vi "Autonomous IndependentAPRIL1st.vi"() -> ()   [LabVIEW 2016]
doc: "This VI is called when autonomous begins, and will automatically be terminated when autonomous ends. You can carry out timed or sensor driven robot movement independently without needing to return to the caller."
uses:
  <vilib>/Rock Robotics/WPI/Utilities/WPI_GetSetVariantRefNum.vi
  <vilib>/Rock Robotics/Network Tables/NT Read String.vi
  <vilib>/Rock Robotics/Network Tables/NT Write Numeric Array.vi
  <vilib>/Rock Robotics/WPI/RobotDrive/WPI_RobotDriveArcadeDrive_Standard(NoSaturation).vi
  <vilib>/Rock Robotics/Network Tables/NT Read Boolean.vi
  <vilib>/Rock Robotics/Network Tables/NT Write Number.vi
  Robot Global Data.vi
  <vilib>/Rock Robotics/WPI/Counter/WPI_CounterDigitalInputToDigitalSource.vi
  <vilib>/Rock Robotics/SystemInterfaces/DIO/FPGA_DIOChannel.ctl
panel:
  out "Hook Center Cons":dbl
  out "gyro":dbl
  out "sonar distance (inches)":dbl
  out "Encoder Loop":dbl
  out "Encoder Loop":string
  out "Current Movement, for debugging 2":T1 {"Y Joystick Value" scale=1.0..-1.0; "X Joystick Value" scale=-1.0..1.0}
  in  "Array of robot movements 2":T2(array[cluster])=[{"X Joystick Value"=0.39393939393939403, "Y Joystick Value"=0.0, "Delay (sec)"=1.0, "Movement Name"="turn"}, {"X Joystick Value"=-0.3737373737373737, "Y Joystick Value"=0.0, "Delay (sec)"=1.0, "Movement Name"="turn back"}] {"Y Joystick Value" scale=1.0..-1.0; "X Joystick Value" scale=-1.0..1.0}
  out "Current Movement, for debugging":T1 {"Y Joystick Value" scale=1.0..-1.0; "X Joystick Value" scale=-1.0..1.0}
  in  "Array of robot movements":T2(array[cluster])=[{"X Joystick Value"=0.39393939393939403, "Y Joystick Value"=0.0, "Delay (sec)"=1.0, "Movement Name"="turn"}, {"X Joystick Value"=-0.3737373737373737, "Y Joystick Value"=0.0, "Delay (sec)"=1.0, "Movement Name"="turn back"}] {"Y Joystick Value" scale=1.0..-1.0; "X Joystick Value" scale=-1.0..1.0}
  # "Sensor Readings\nConstanly updated in\nwhile loopes"
  # "Be sure to right-click and choose Data Operations>>Make Current Value default if you want to save the array values with the VI"
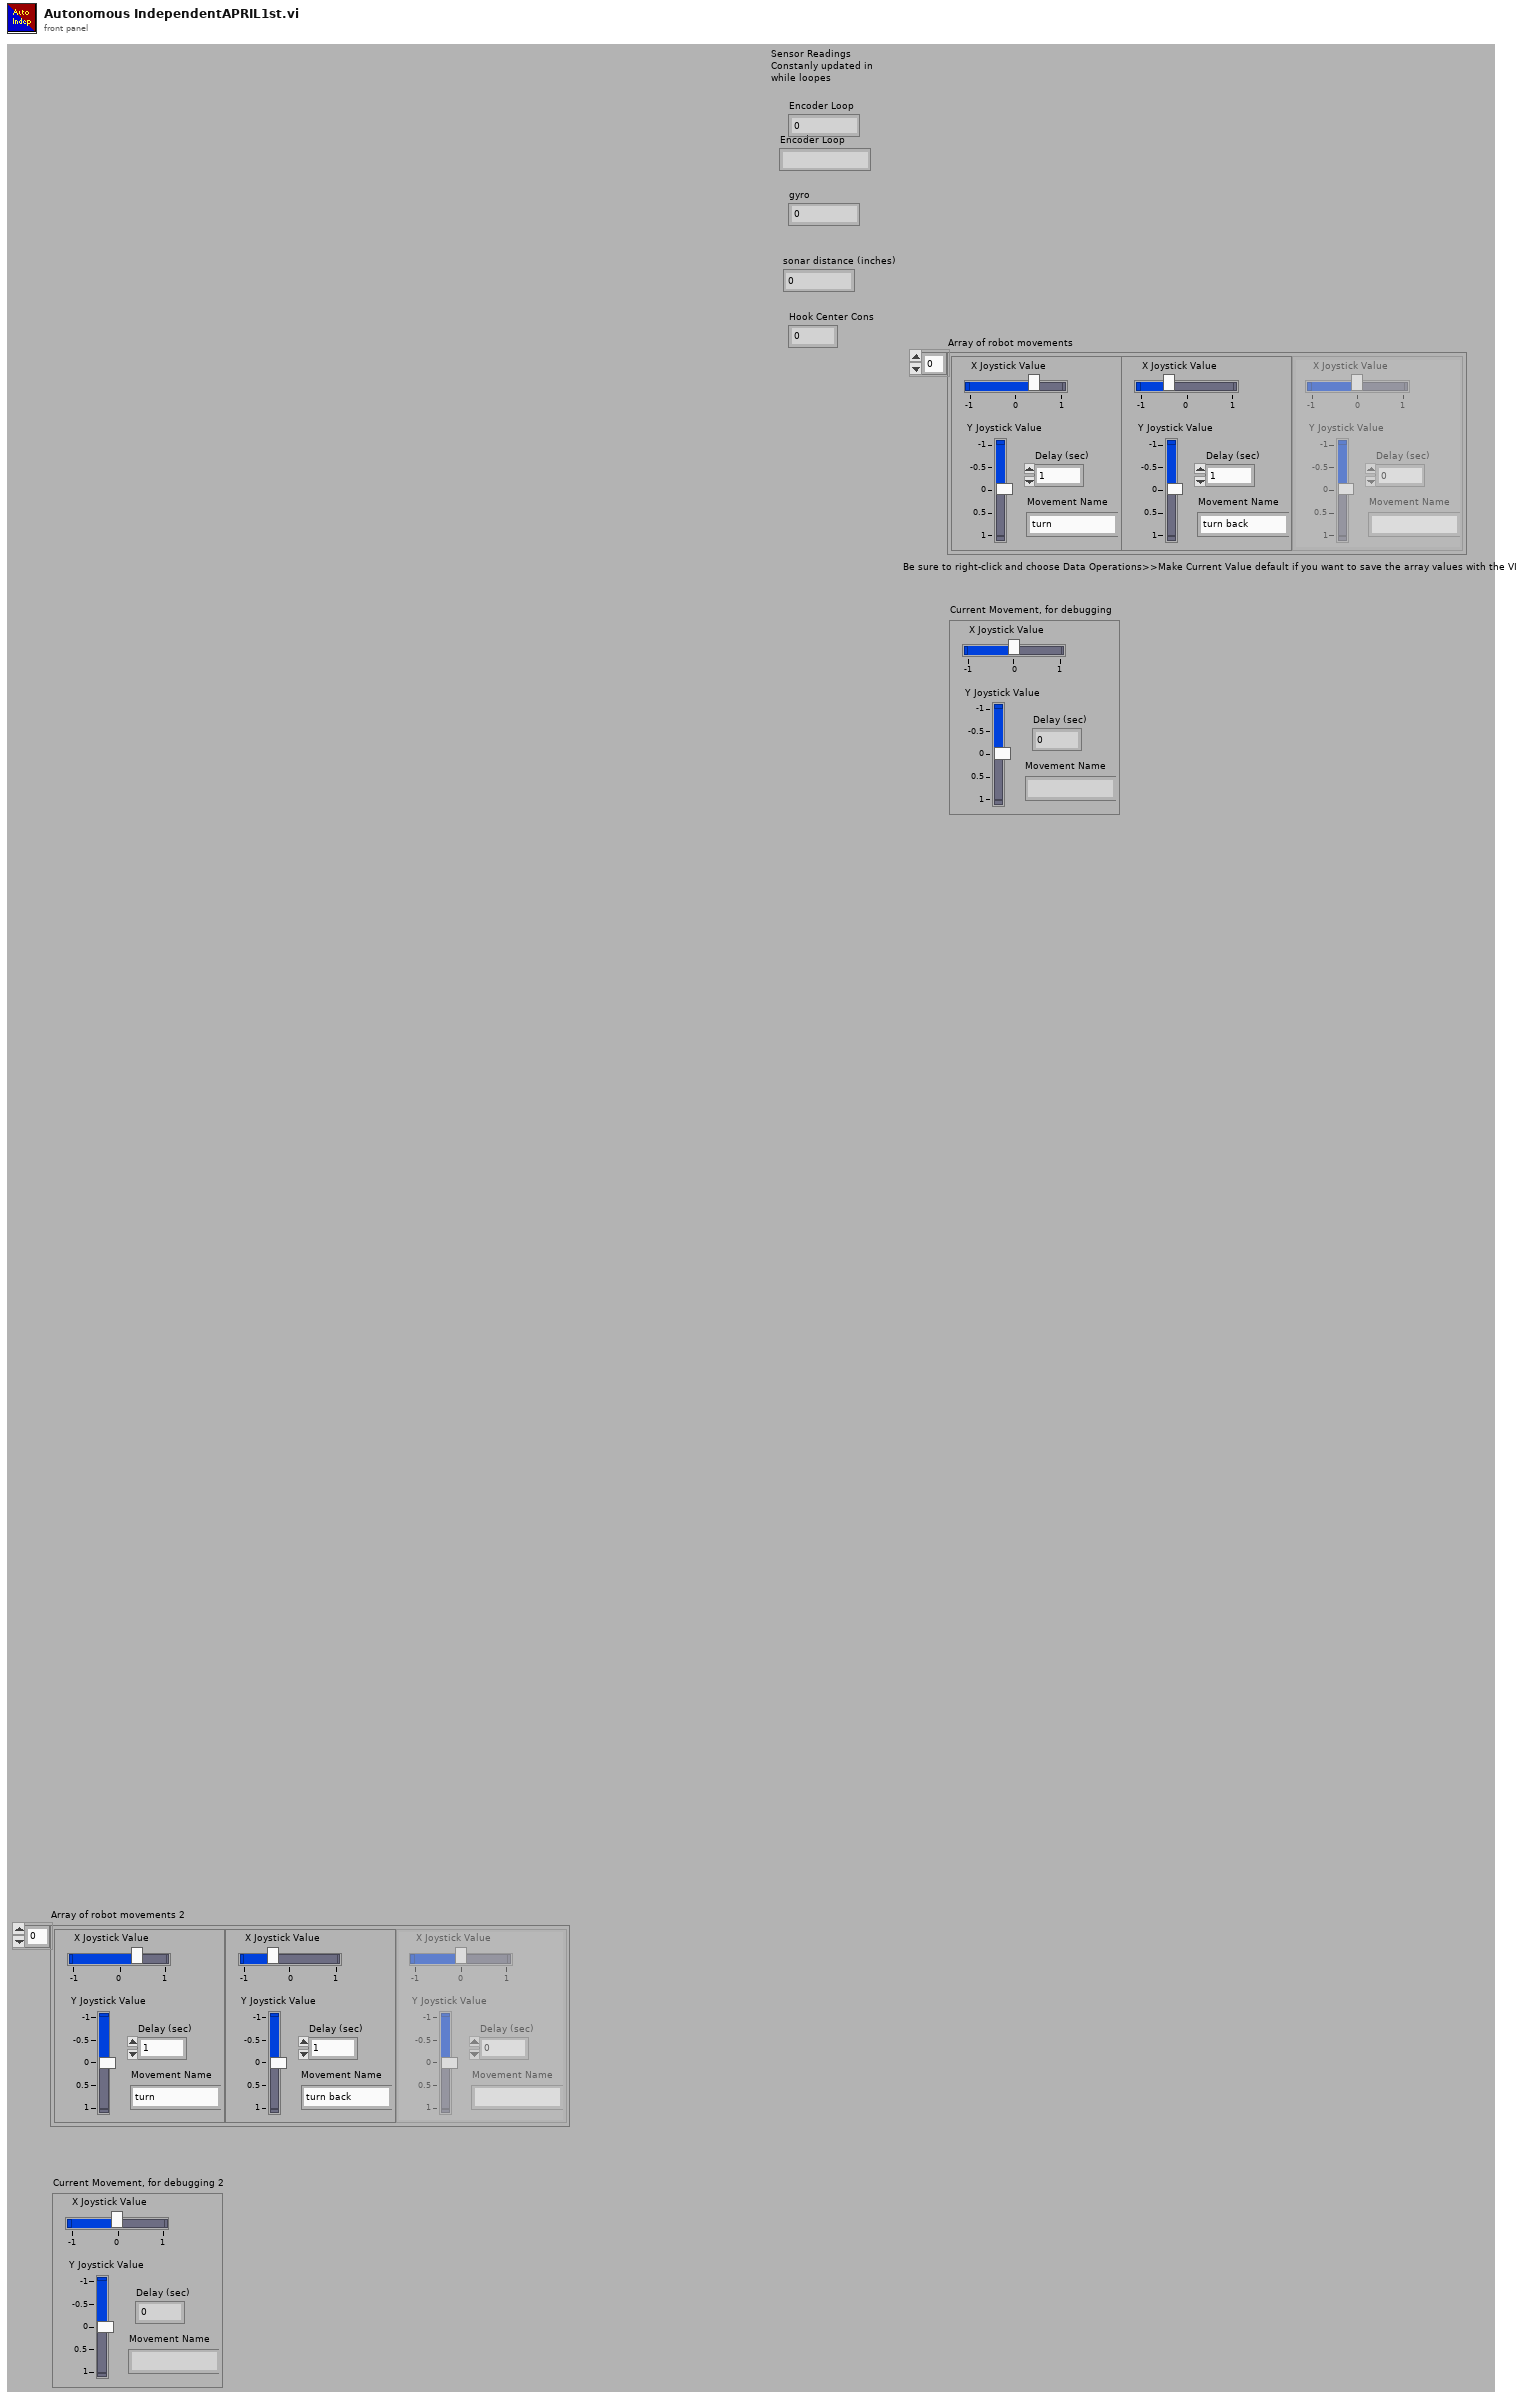
[diagram p1: front panel]
types:
  T1 = cluster{"X Joystick Value":dbl, "Y Joystick Value":dbl, "Delay (sec)":dbl, "Movement Name":string}
  T2 = cluster{"X Joystick Value":dbl, "Y Joystick Value":dbl, "Delay (sec)":dbl, "Movement Name":string}[]
  T3 = typedef "FPGA_DIOChannel.ctl" = enum8{"DIO 0", "DIO 1", "DIO 2", "DIO 3", "DIO 4", "DIO 5", "DIO 6", "DIO 7", "DIO 8", "DIO 9", "DIO MXP 0", "DIO MXP 1", "DIO MXP 2", "DIO MXP 3", "DIO MXP 4", "DIO MXP 5", "DIO MXP 6", "DIO MXP 7", "DIO MXP 8", "DIO MXP 9", "DIO MXP 10", "DIO MXP 11", "DIO MXP 12", "DIO MXP 13", "DIO MXP 14", "DIO MXP 15", "SPI Port CS1", "SPI Port CS2", "SPI Port CS3", "SPI Port MISO", "SPI Port MOSI", "Invalid"}
  T4 = typedef "WPI_DigitalInputDevRef.ctl" = cluster{"DevStatus":errorcluster, "DIO Channel":T3}
  T5 = typedef "FPGA_CounterEncoderSourceConvertionLVSourceType.ctl" = cluster{"DevStatus":errorcluster, "AnalogTriggerMode?":bool, "DigitalMode":cluster{"DIO Channel":T6}, "AnalogTriggerMode":cluster{"AnalogTriggerIndex":T7, "OutputType":T8}}
  T6 = typedef "FPGA_DIODigitalSourceChannel.ctl" = enum8{"DIO 0", "DIO 1", "DIO 2", "DIO 3", "DIO 4", "DIO 5", "DIO 6", "DIO 7", "DIO 8", "DIO 9", "DIO MXP 0", "DIO MXP 1", "DIO MXP 2", "DIO MXP 3", "DIO MXP 4", "DIO MXP 5", "DIO MXP 6", "DIO MXP 7", "DIO MXP 8", "DIO MXP 9", "DIO MXP 10", "DIO MXP 11", "DIO MXP 12", "DIO MXP 13", "DIO MXP 14", "DIO MXP 15", "Disabled"}
  T7 = typedef "FPGA_AnalogTriggerIndex.ctl" = enum8{"Trig 0", "Trig 1", "Trig 2", "Trig 3", "Trig 4", "Trig 5", "Trig 6", "Trig 7", "Invalid"}
  T8 = typedef "FPGA_AnalogTriggerOutType.ctl" = enum16{"InWindow", "TriggerState", "Rising", "Falling"}
  T9 = typedef "WPI_EncoderDevRef.ctl" = cluster{"DevStatus":errorcluster, "EncoderIndex":T10, "CounterIndex":T11, "DistancePerCount":dbl, "Decoding Type":T12}
  T10 = typedef "FPGA_EncoderIdx.ctl" = enum8{"Enc 0", "Enc 1", "Enc 2", "Enc 3", "Enc 4", "Enc 5", "Enc 6", "Enc 7", "Invalid"}
  T11 = typedef "FPGA_CounterCtrSystemIndex.ctl" = enum8{"Ctr 0", "Ctr 1", "Ctr 2", "Ctr 3", "Ctr 4", "Ctr 5", "Ctr 6", "Ctr 7", "Invalid"}
  T12 = typedef "WPI_EncoderType.ctl" = enum16{"1x", "2x", "4x"}
  T13 = typedef "WPI_JoystickDevRef.ctl" = cluster{"Device":T14}
  T14 = typedef "WPI_JoystickDeviceEnum.ctl" = enum16{"USB 0", "USB 1", "USB 2", "USB 3", "USB 4", "USB 5"}
  T15 = typedef "WPI_DriverStationPositionInfo.ctl" = enum16{"1", "2", "3"}
  T16 = typedef "WPI_RobotDriveDevRef.ctl" = cluster{"DevStatus":errorcluster, "Motors[]":T17[], "Square Inputs":bool, "Max Output":dbl}
  T17 = typedef "WPI_MotorControlDeviceRef.ctl" = cluster{"DeviceStatus":errorcluster, "Type":T18, "PWM":cluster{"PWM Channel":T19, "DeadBand":T20}, "CAN":cluster{"Device Number":u8, "SetOutput VI Ref":variant, "GetOutput VI Ref":variant, "Enable VI Ref":variant, "Disable VI Ref":variant, "Data":variant}, "Invert":bool}
  T18 = typedef "WPI_MotorControlType.ctl" = enum16{"PWM", "CAN"}
  T19 = typedef "FPGA_DIOPWMChannel.ctl" = enum8{"PWM 0", "PWM 1", "PWM 2", "PWM 3", "PWM 4", "PWM 5", "PWM 6", "PWM 7", "PWM 8", "PWM 9", "PWM MXP 0", "PWM MXP 1", "PWM MXP 2", "PWM MXP 3", "PWM MXP 4", "PWM MXP 5", "PWM MXP 6", "PWM MXP 7", "PWM MXP 8", "PWM MXP 9", "Invalid"}
  T20 = typedef "WPI_PWMDeadband.ctl" = cluster{"Name":string, "maxPositivePwm":i32, "minPositivePwm":i32, "centerPwm":i32, "maxNegativePwm":i32, "minNegativePwm":i32, "angularRange":u16}
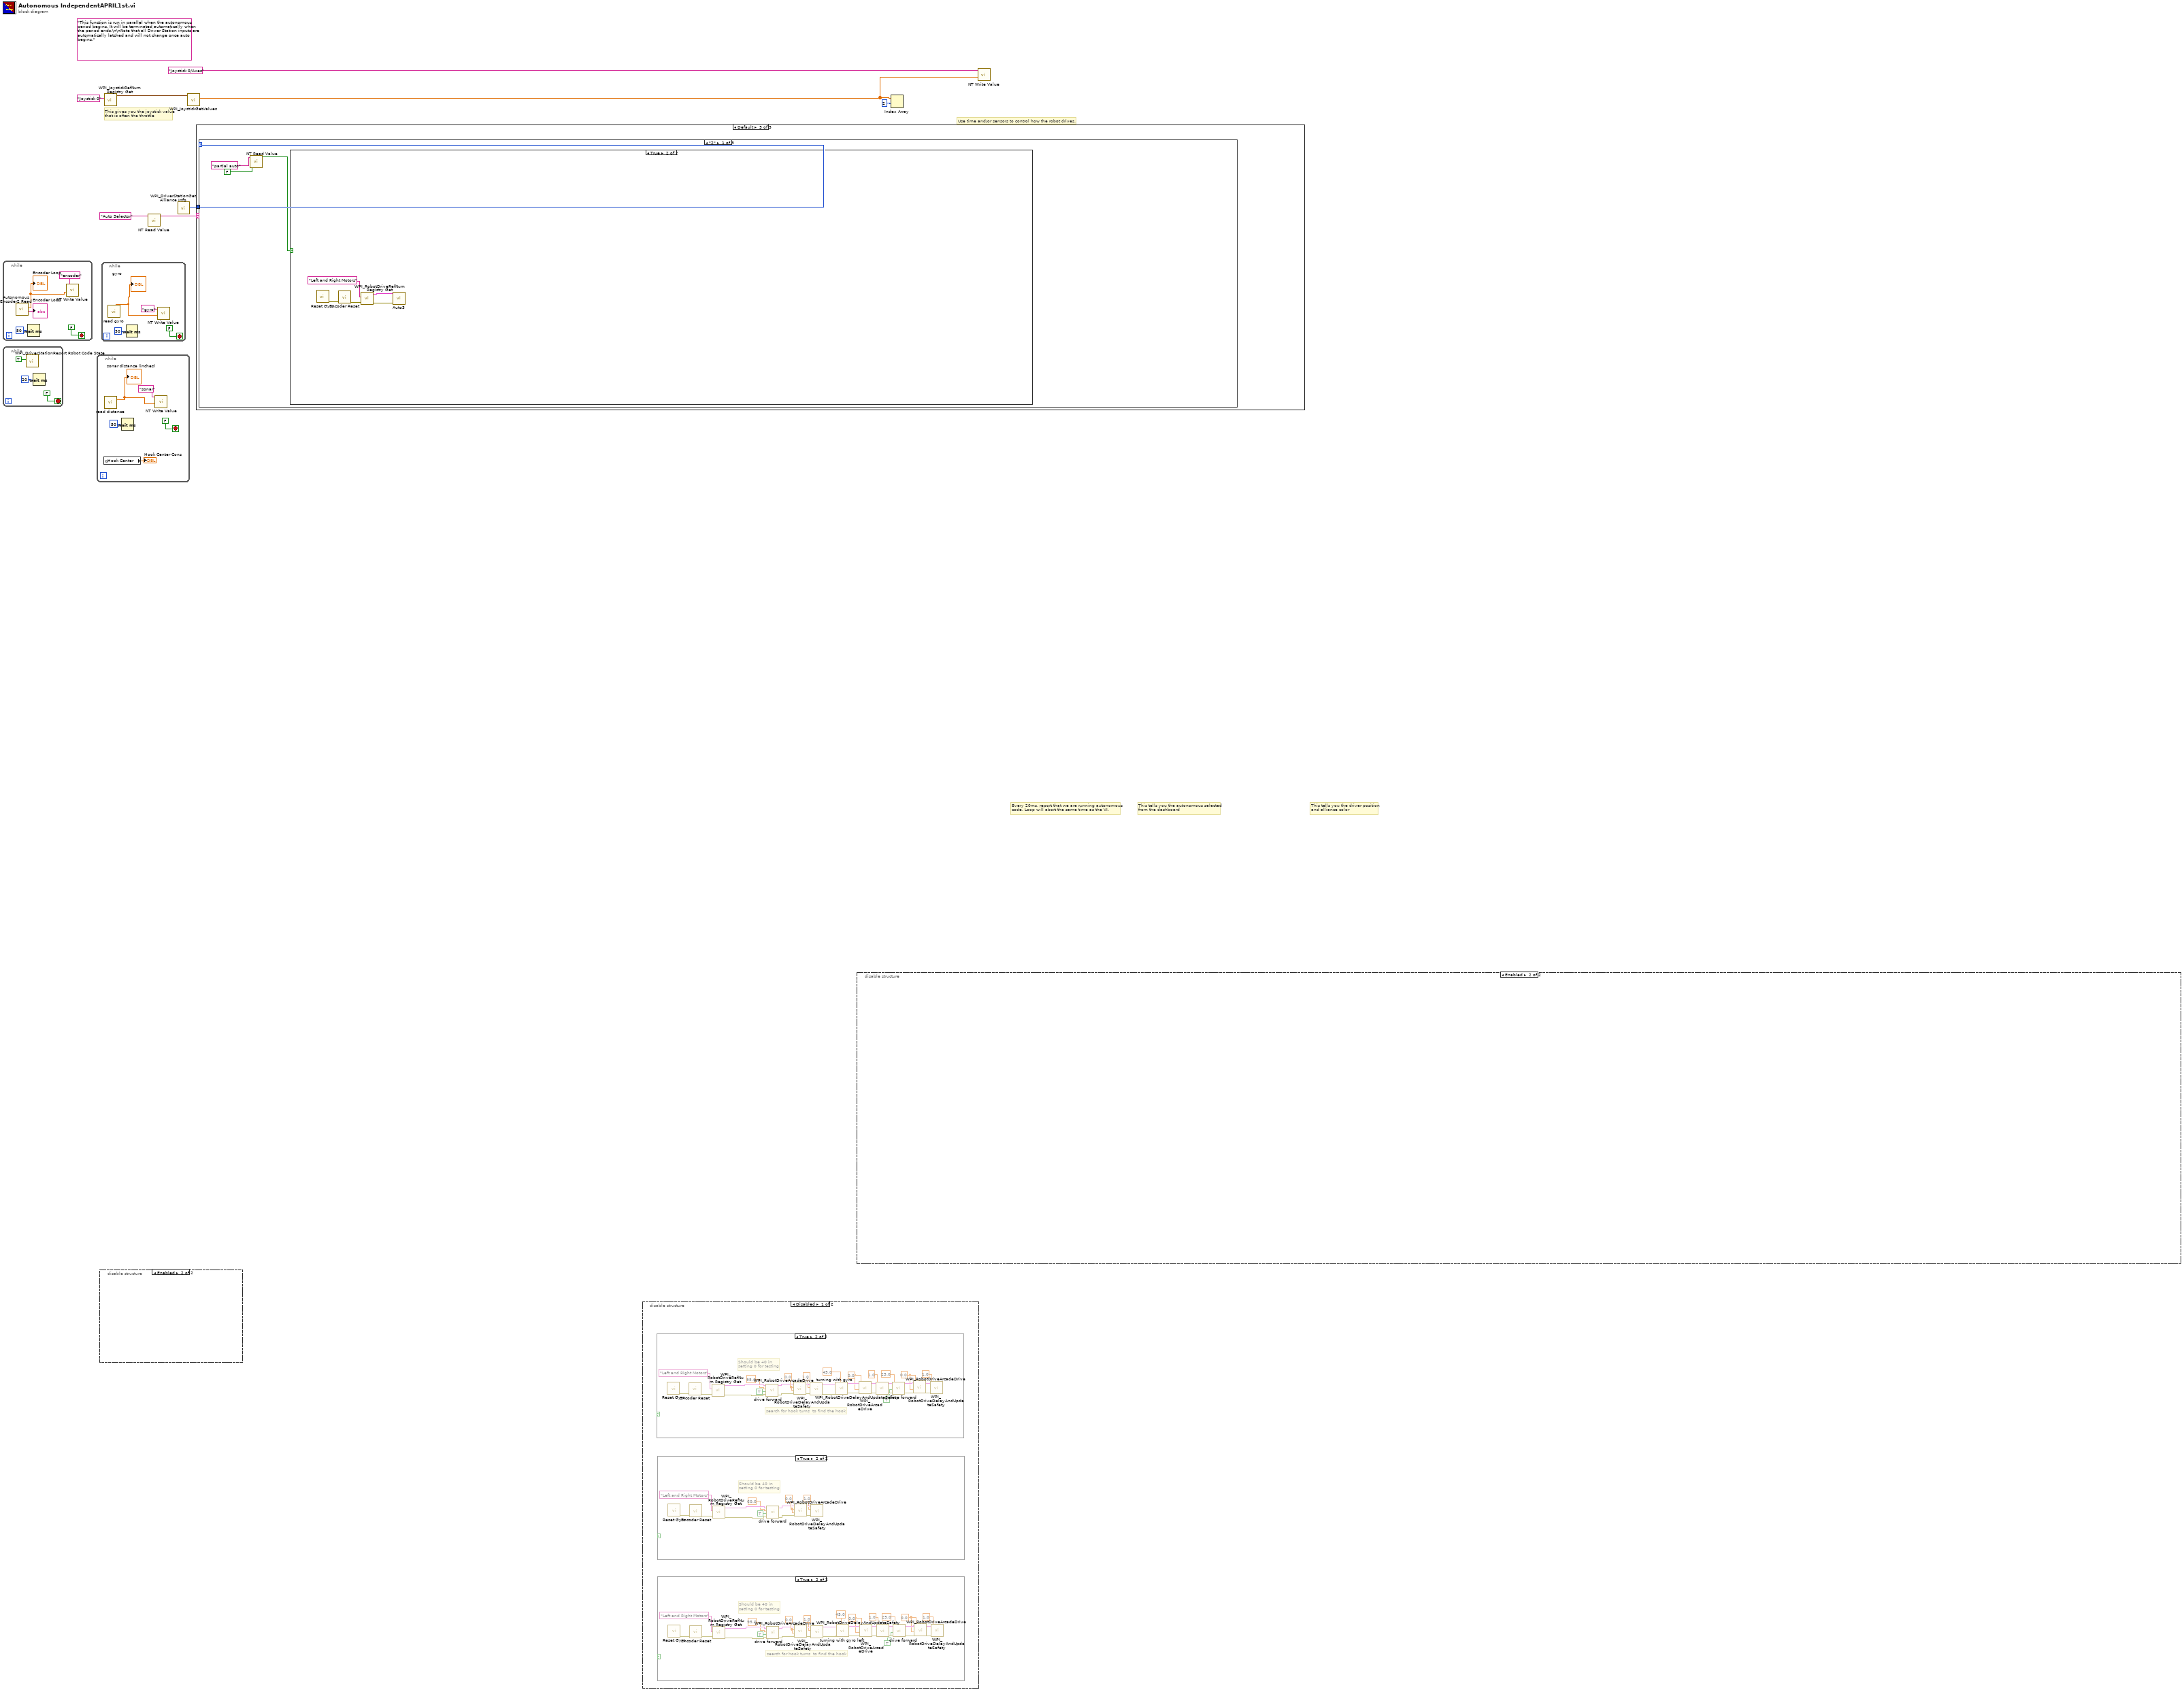
[diagram p0: block diagram]
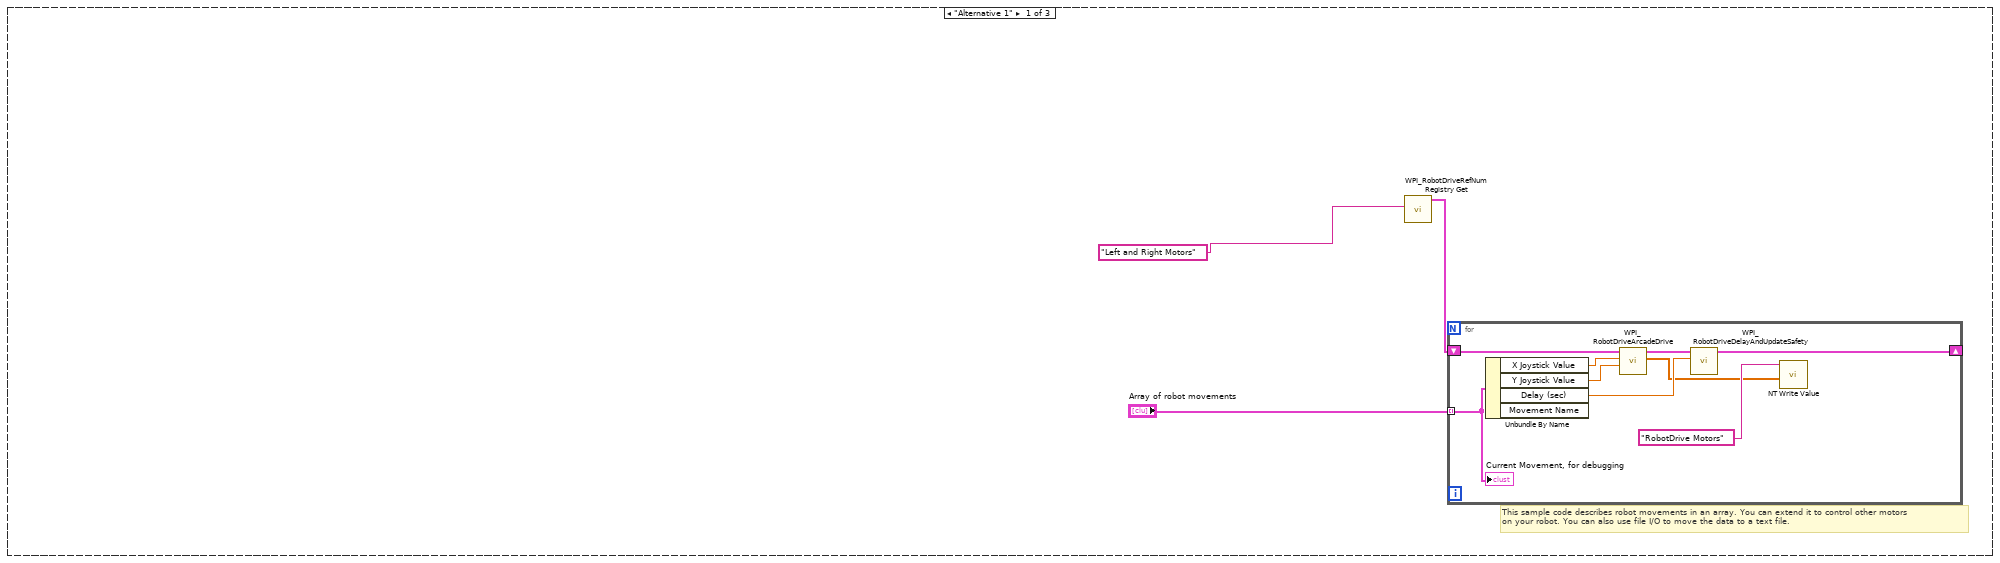
[diagram p6: hidden frame]
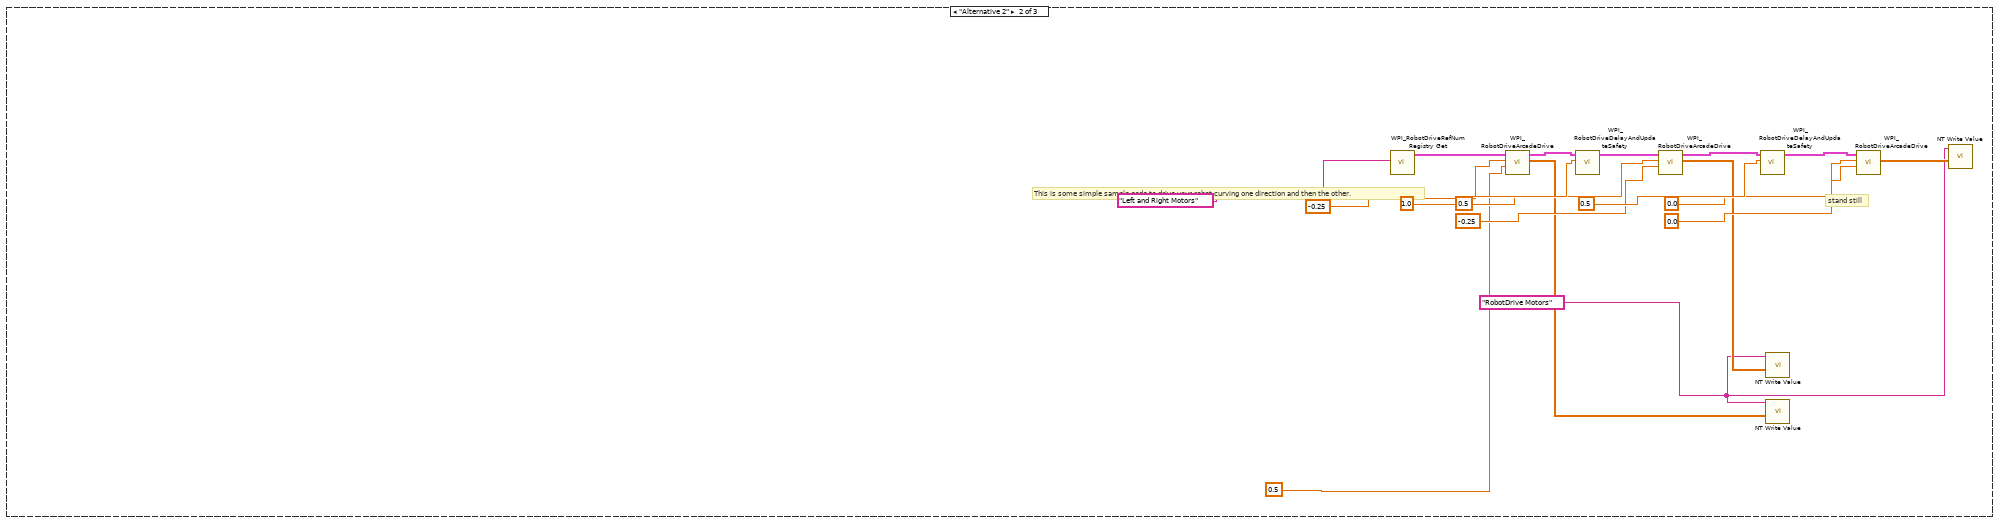
[diagram p7: hidden frame]
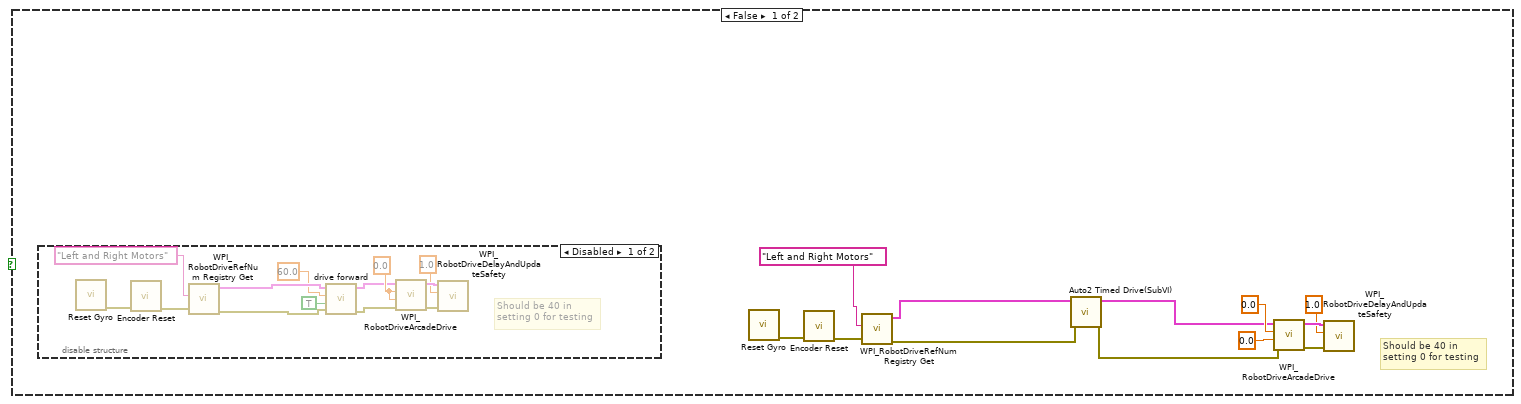
[diagram p8: hidden frame]
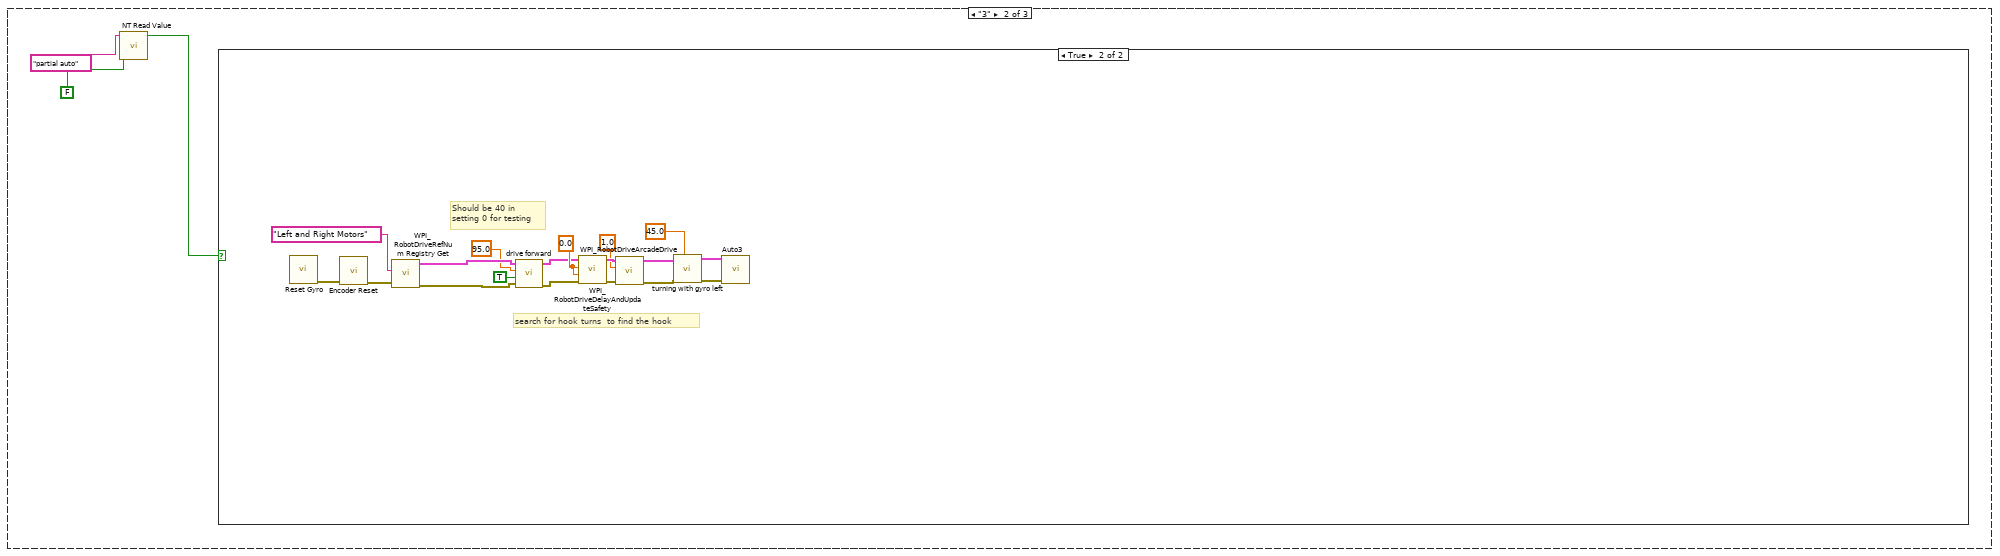
[diagram p10: hidden frame]
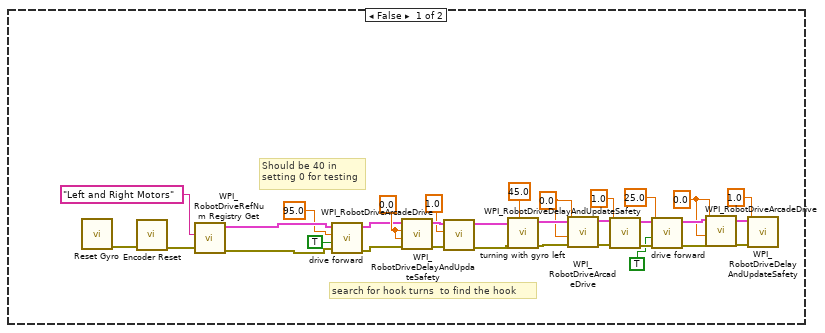
[diagram p11: hidden frame]
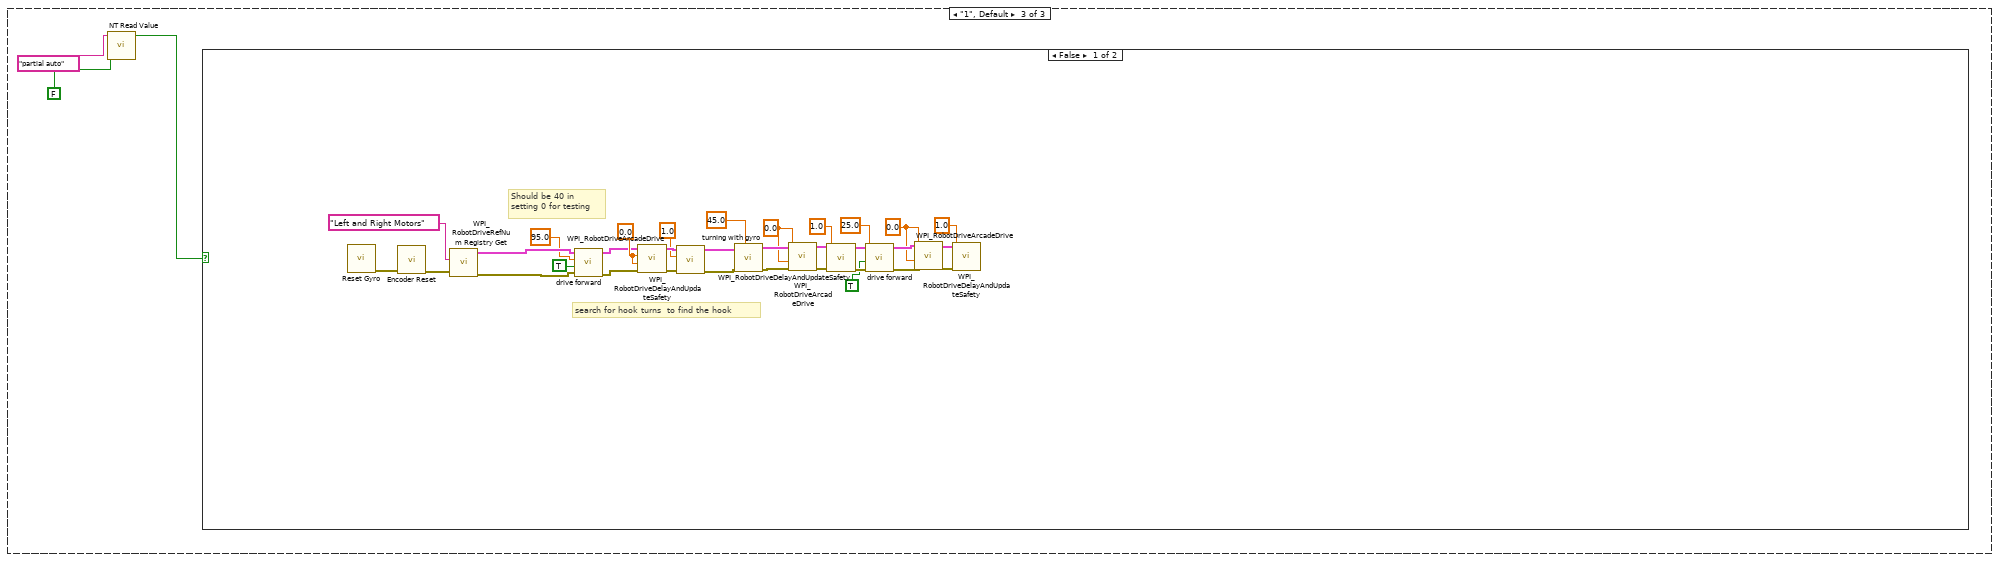
[diagram p12: hidden frame]
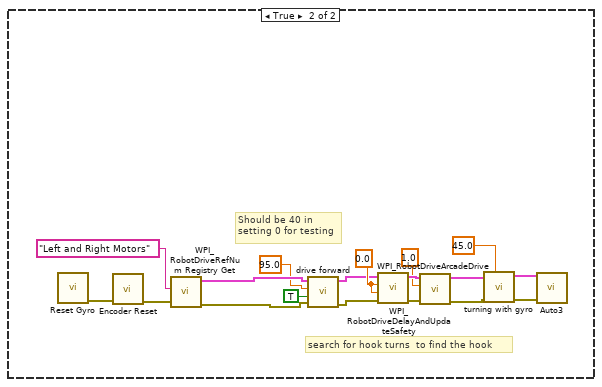
[diagram p13: hidden frame]
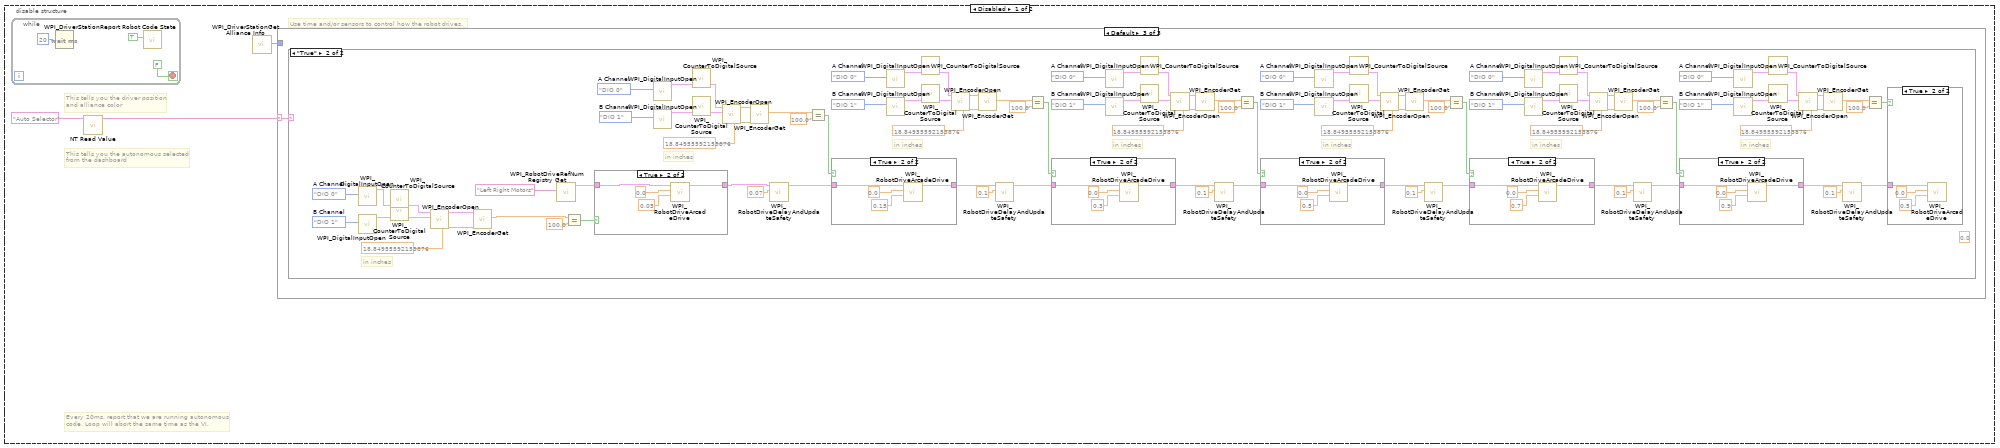
[diagram p14: hidden frame]
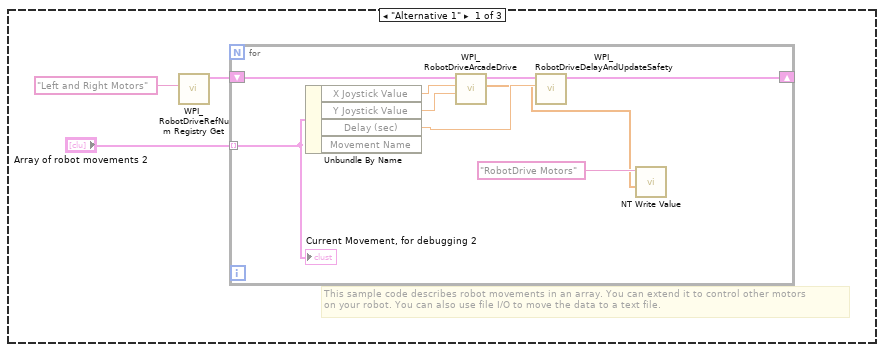
[diagram p15: hidden frame]
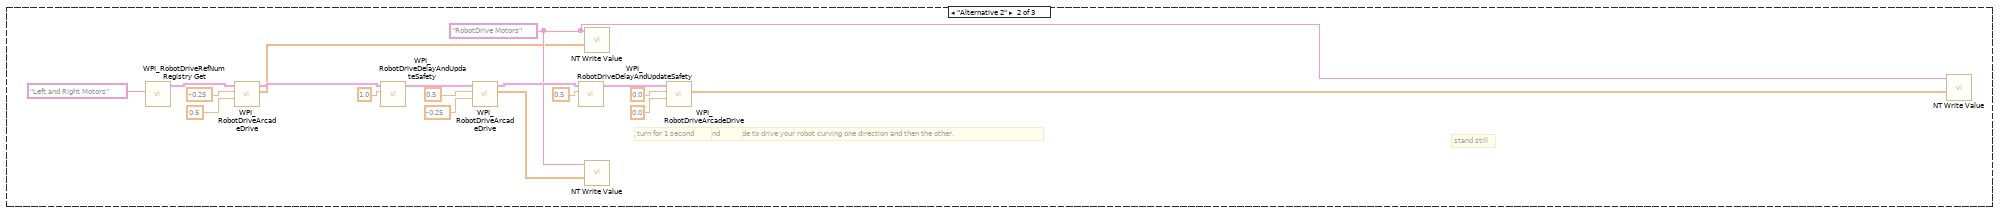
[diagram p16: hidden frame]
diagram:
  (unwired) "This function is run in parallel when the autonomous period begins. It will be terminated automatically when the period ends.\n\nNote that all Driver Station inputs are automatically latched and will not change once auto begins."
  # "This tells you the autonomous selected\nfrom the dashboard"
  # "Every 20ms, report that we are running autonomous\ncode. Loop will abort the same time as the VI."
  # "This gives you the joystick value\nthat is often the throttle"
  # "Use time and/or sensors to control how the robot drives."
  # "This tells you the driver position\nand alliance color"
  n1 = while {
    stop <- FALSE stop-if-true
    n2 = call "Autonomous Encoder2 Read.vi"() -> ("Encoder Direction"=→"Encoder Loop":string, "Encoder Distance"=w10:dbl)  [unwired: 9 in, 1 out]
    "Encoder Loop" <- w10
    n3 = Wait (ms)(milliseconds to wait=u32 50) -> ()  [unwired: 1 out]
    n4 = call-poly <vilib>:"NT Write Value.vi"("Numeric"=w10, "Name"="encoder") -> ()  [unwired: 9 in, 1 out]
  }
  n5 = while {
    stop <- FALSE stop-if-true
    n6 = call <vilib>:"WPI_DriverStationReport Robot Code State.vi"("Autonomous"=TRUE) -> ()  [unwired: 10 in, 1 out]
    n7 = Wait (ms)(milliseconds to wait=u32 20) -> ()  [unwired: 1 out]
  }
  n8 = while {
    stop <- FALSE stop-if-true
    n9 = global read "Robot Global Data.vi" "Hook Center"() -> (→"Hook Center Cons":dbl)
    n10 = call "read distance.vi"() -> ("Distance 2"=w19:dbl)  [unwired: 10 in, 1 out]
    "sonar distance (inches)" <- w19
    n11 = Wait (ms)(milliseconds to wait=u32 50) -> ()  [unwired: 1 out]
    n12 = call-poly <vilib>:"NT Write Value.vi"("Numeric"=w19, "Name"="sonar") -> ()  [unwired: 9 in, 1 out]
  }
  n13 = disable-structure shown="Enabled" {
    frame Disabled {
      w35 = FPGA_DIOChannel."DIO 1"  # B Channel
      w34 = FPGA_DIOChannel."DIO 0"  # A Channel
      # "in inches"
      n14 = call <vilib>:"WPI_DigitalInputOpen.vi"("DIO Channel"=w34) -> ("DigitalInputDevRef"=w31:T4)  [unwired: 1 in, 9 out]
      n15 = call <vilib>:"WPI_DigitalInputOpen.vi"("DIO Channel"=w35) -> ("DigitalInputDevRef"=w32:T4)  [unwired: 1 in, 9 out]
      n16 = call-poly <vilib>:"WPI_CounterToDigitalSource.vi"("DigitalInputDevRef"=w31) -> ("Digital Source"=w30:T5)  [unwired: 6 out]
      n17 = call-poly <vilib>:"WPI_CounterToDigitalSource.vi"("DigitalInputDevRef"=w32) -> ("Digital Source"=w33:T5)  [unwired: 6 out]
      n18 = call <vilib>:"WPI_EncoderOpen.vi"("DistancePerCount"=18.84955592153876, "Invert Direction (False)"=FALSE, "BSource"=w33, "ASource"=w30) -> ("error out"=w28:errorcluster, "EncoderDevRef"=w29:T9)  [unwired: 4 in, 2 out]
      n19 = call-poly <vilib>:"NT Write Value.vi"("Name"="Encoder Distance") -> ()  [unwired: 10 in, 1 out]
      n20 = call <vilib>:"WPI_EncoderRefNum Registry Set.vi"("error in (no error)"=w28, "refnum name"="Encoder", "EncoderDevRef"=w29) -> ("error out"=w26:errorcluster, "EncoderDevRef"=w27:T9)  [unwired: 7 in]
      n21 = call <vilib>:"WPI_EncoderGet.vi"("error in (no error)"=w26, "EncoderDevRef"=w27) -> ()  [unwired: 4 in, 6 out]
    }
    frame Enabled {
    }
  }
  n22 = while {
    stop <- FALSE stop-if-true
    n23 = call "read gyro.vi"() -> ("Angle 2"=w37:dbl)  [unwired: 10 in, 1 out]
    "gyro" <- w37
    n24 = Wait (ms)(milliseconds to wait=u32 50) -> ()  [unwired: 1 out]
    n25 = call-poly <vilib>:"NT Write Value.vi"("Numeric"=w37, "Name"="gyro") -> ()  [unwired: 9 in, 1 out]
  }
  n26 = call <vilib>:"WPI_JoystickRefNum Registry Get.vi"("refnum name"="Joystick 0") -> ("JoystickDevRef"=w7:T13)  [unwired: 1 in, 9 out]
  n27 = call-poly <vilib>:"NT Read Value.vi"("Name"="Auto Selector") -> ("String"=w4:string)  [unwired: 9 in, 1 out]
  n28 = call <vilib>:"WPI_DriverStationGet Alliance Info.vi"() -> ("Position"=w1:T15)  [unwired: 11 out]
  n29 = call <vilib>:"WPI_JoystickGetValues.vi"("JoystickDevRef"=w7) -> ("Axes"=w3:dbl[])  [unwired: 6 in, 4 out]
  n30 = case shown="Default" w4 {
    tunnel: w1 -> [_ _ w70]
    frame "Alternative 1" {
      # "This sample code describes robot movements in an array. You can extend it to control other motors\non your robot. You can also use file I/O to move the data to a text file."
      n31 = call <vilib>:"WPI_RobotDriveRefNum Registry Get.vi"("refnum name"="Left and Right Motors") -> ("RobotDriveDevRef"=w41:T16)  [unwired: 1 in, 9 out]
      n32 = for {
        shift-right: [w49] -> _
        shift-left: w41 -> [w50]
        tunnel: "Array of robot movements" -> [w45] mode=indexing
        n33 = Unbundle By Name(w45) -> ("X Joystick Value"=w48:dbl, "Y Joystick Value"=w47:dbl, "Delay (sec)"=w46:dbl)  [unwired: 1 out]
        n34 = call-poly <vilib>:"WPI_RobotDriveArcadeDrive.vi"("Y axis value"=w47, "X axis value"=w48, "RobotDriveDevRef"=w50) -> ("Motor Values"=w43:dbl[], "RobotDriveDevRef"=w51:T16)  [unwired: 1 in, 6 out]
        n35 = call <vilib>:"WPI_RobotDriveDelayAndUpdateSafety.vi"("Delay (s)"=w46, "RobotDriveDevRef"=w51) -> ("RobotDriveDevRef 2"=w49:T16)  [unwired: 8 in, 1 out]
        n36 = call-poly <vilib>:"NT Write Value.vi"("Numeric Array"=w43, "Name"="RobotDrive Motors") -> ()  [unwired: 9 in, 1 out]
        "Current Movement, for debugging" <- w45
      }
    }
    frame "Alternative 2" {
      w53 = "RobotDrive Motors" ("Name")
      # "This is some simple sample code to drive your robot curving one direction and then the other."
      # "stand still"
      n37 = call <vilib>:"WPI_RobotDriveRefNum Registry Get.vi"("refnum name"="Left and Right Motors") -> ("RobotDriveDevRef"=w69:T16)  [unwired: 1 in, 9 out]
      n38 = call-poly <vilib>:"WPI_RobotDriveArcadeDrive.vi"("Y axis value"=0.5 ("X axis value"), "X axis value"=-0.25, "RobotDriveDevRef"=w69) -> ("Motor Values"=w52:dbl[], "RobotDriveDevRef"=w62:T16)  [unwired: 1 in, 6 out]
      n39 = call <vilib>:"WPI_RobotDriveDelayAndUpdateSafety.vi"("Delay (s)"=1.0, "RobotDriveDevRef"=w62) -> ("RobotDriveDevRef 2"=w63:T16)  [unwired: 8 in, 1 out]
      n40 = call-poly <vilib>:"WPI_RobotDriveArcadeDrive.vi"("Y axis value"=-0.25 ("X axis value"), "X axis value"=0.5, "RobotDriveDevRef"=w63) -> ("Motor Values"=w54:dbl[], "RobotDriveDevRef"=w64:T16)  [unwired: 1 in, 6 out]
      n41 = call <vilib>:"WPI_RobotDriveDelayAndUpdateSafety.vi"("Delay (s)"=0.5, "RobotDriveDevRef"=w64) -> ("RobotDriveDevRef 2"=w65:T16)  [unwired: 8 in, 1 out]
      n42 = call-poly <vilib>:"NT Write Value.vi"("Numeric Array"=w54, "Name"=w53) -> ()  [unwired: 9 in, 1 out]
      n43 = call-poly <vilib>:"NT Write Value.vi"("Numeric Array"=w52, "Name"=w53) -> ()  [unwired: 9 in, 1 out]
      n44 = call-poly <vilib>:"WPI_RobotDriveArcadeDrive.vi"("Y axis value"=0.0 ("X axis value"), "X axis value"=0.0, "RobotDriveDevRef"=w65) -> ("Motor Values"=w55:dbl[])  [unwired: 1 in, 7 out]
      n45 = call-poly <vilib>:"NT Write Value.vi"("Numeric Array"=w55, "Name"=w53) -> ()  [unwired: 9 in, 1 out]
    }
    frame Default {
      n46 = case shown="\"2\"" w70 {
        frame "2" {
          n47 = call-poly <vilib>:"NT Read Value.vi"("Default Value"=FALSE, "Name"="partial auto") -> ("Boolean"=w71:bool)  [unwired: 8 in, 1 out]
          n48 = case shown="True" w71 {
            frame False {
              # "Should be 40 in\nsetting 0 for testing"
              n49 = disable-structure shown="Disabled" {
                frame Disabled {
                  w88 = 0.0 ("X axis value")
                  # "Should be 40 in\nsetting 0 for testing"
                  n50 = call "Reset Gyro.vi"() -> ("error out"=w95:errorcluster)  [unwired: 11 in]
                  n51 = call "Encoder Reset.vi"("error in (no error)"=w95) -> ("error out"=w97:errorcluster)  [unwired: 10 in]
                  n52 = call <vilib>:"WPI_RobotDriveRefNum Registry Get.vi"("error in (no error)"=w97, "refnum name"="Left and Right Motors") -> ("error out"=w94:errorcluster, "RobotDriveDevRef"=w96:T16)  [unwired: 8 out]
                  n53 = call "drive forward.vi"("error in (no error)"=w94, "forward"=TRUE, "desired distance"=60.0, "RobotDriveDevRef in"=w96) -> ("error out"=w86:errorcluster, "RobotDriveDevRef out"=w87:T16)  [unwired: 6 in]
                  n54 = call-poly <vilib>:"WPI_RobotDriveArcadeDrive.vi"("error in (no error)"=w86, "Y axis value"=w88, "X axis value"=w88, "RobotDriveDevRef"=w87) -> ("error out"=w90:errorcluster, "RobotDriveDevRef"=w91:T16)  [unwired: 6 out]
                  n55 = call <vilib>:"WPI_RobotDriveDelayAndUpdateSafety.vi"("error in (no error)"=w90, "Delay (s)"=1.0, "RobotDriveDevRef"=w91) -> ()  [unwired: 7 in, 2 out]
                }
                frame Enabled {
                }
              }
              n56 = call "Reset Gyro.vi"() -> ("error out"=w84:errorcluster)  [unwired: 11 in]
              n57 = call "Encoder Reset.vi"("error in (no error)"=w84) -> ("error out"=w85:errorcluster)  [unwired: 10 in]
              n58 = call <vilib>:"WPI_RobotDriveRefNum Registry Get.vi"("error in (no error)"=w85, "refnum name"="Left and Right Motors") -> ("error out"=w78:errorcluster, "RobotDriveDevRef"=w79:T16)  [unwired: 8 out]
              n59 = call "Auto2 Timed Drive(SubVI).vi"("error in (no error)"=w78, "RobotDriveDevRef in"=w79) -> ("error out"=w74:errorcluster, "RobotDriveDevRef out"=w75:T16)  [unwired: 8 in]
              n60 = call-poly <vilib>:"WPI_RobotDriveArcadeDrive.vi"("error in (no error)"=w74, "Y axis value"=0.0, "X axis value"=0.0, "RobotDriveDevRef"=w75) -> ("error out"=w82:errorcluster, "RobotDriveDevRef"=w83:T16)  [unwired: 6 out]
              n61 = call <vilib>:"WPI_RobotDriveDelayAndUpdateSafety.vi"("error in (no error)"=w82, "Delay (s)"=1.0, "RobotDriveDevRef"=w83) -> ()  [unwired: 7 in, 2 out]
            }
            frame True {
              n62 = call "Reset Gyro.vi"() -> ("error out"=w100:errorcluster)  [unwired: 11 in]
              n63 = call "Encoder Reset.vi"("error in (no error)"=w100) -> ("error out"=w102:errorcluster)  [unwired: 10 in]
              n64 = call <vilib>:"WPI_RobotDriveRefNum Registry Get.vi"("error in (no error)"=w102, "refnum name"="Left and Right Motors") -> ("error out"=w99:errorcluster, "RobotDriveDevRef"=w101:T16)  [unwired: 8 out]
              n65 = call "Auto3.vi"("RobotDriveDevRef"=w101, "error in (no error)"=w99) -> ()  [unwired: 6 in, 8 out]
            }
          }
        }
        frame "3" {
          n66 = call-poly <vilib>:"NT Read Value.vi"("Default Value"=FALSE, "Name"="partial auto") -> ("Boolean"=w104:bool)  [unwired: 8 in, 1 out]
          n67 = case shown="True" w104 {
            frame False {
              w110 = 0.0 ("X axis value")
              w121 = 0.0 ("X axis value")
              w128 = 0.0 ("X axis value")
              # "search for hook turns  to find the hook"
              # "Should be 40 in\nsetting 0 for testing"
              n68 = call "Reset Gyro.vi"() -> ("error out"=w135:errorcluster)  [unwired: 11 in]
              n69 = call "Encoder Reset.vi"("error in (no error)"=w135) -> ("error out"=w137:errorcluster)  [unwired: 10 in]
              n70 = call <vilib>:"WPI_RobotDriveRefNum Registry Get.vi"("error in (no error)"=w137, "refnum name"="Left and Right Motors") -> ("error out"=w134:errorcluster, "RobotDriveDevRef"=w136:T16)  [unwired: 8 out]
              n71 = call "drive forward.vi"("error in (no error)"=w134, "forward"=TRUE, "desired distance"=95.0, "RobotDriveDevRef in"=w136) -> ("error out"=w126:errorcluster, "RobotDriveDevRef out"=w127:T16)  [unwired: 6 in]
              n72 = call-poly <vilib>:"WPI_RobotDriveArcadeDrive.vi"("error in (no error)"=w126, "Y axis value"=w128, "X axis value"=w128, "RobotDriveDevRef"=w127) -> ("error out"=w130:errorcluster, "RobotDriveDevRef"=w131:T16)  [unwired: 6 out]
              n73 = call <vilib>:"WPI_RobotDriveDelayAndUpdateSafety.vi"("error in (no error)"=w130, "Delay (s)"=1.0, "RobotDriveDevRef"=w131) -> ("error out"=w124:errorcluster, "RobotDriveDevRef 2"=w125:T16)  [unwired: 7 in]
              n74 = call "turning with gyro left.vi"("desired angle"=45.0, "error in (no error)"=w124, "RobotDriveDevRef"=w125) -> ("error out"=w118:errorcluster, "RobotDriveDevRef 2"=w122:T16)  [unwired: 7 in]
              n75 = call-poly <vilib>:"WPI_RobotDriveArcadeDrive.vi"("error in (no error)"=w118, "Y axis value"=w121, "X axis value"=w121, "RobotDriveDevRef"=w122) -> ("error out"=w119:errorcluster, "RobotDriveDevRef"=w120:T16)  [unwired: 6 out]
              n76 = call <vilib>:"WPI_RobotDriveDelayAndUpdateSafety.vi"("error in (no error)"=w119, "Delay (s)"=1.0, "RobotDriveDevRef"=w120) -> ("error out"=w116:errorcluster, "RobotDriveDevRef 2"=w115:T16)  [unwired: 7 in]
              n77 = call "drive forward.vi"("error in (no error)"=w116, "forward"=TRUE, "desired distance"=25.0, "RobotDriveDevRef in"=w115) -> ("error out"=w111:errorcluster, "RobotDriveDevRef out"=w112:T16)  [unwired: 6 in]
              n78 = call-poly <vilib>:"WPI_RobotDriveArcadeDrive.vi"("error in (no error)"=w111, "Y axis value"=w110, "X axis value"=w110, "RobotDriveDevRef"=w112) -> ("error out"=w108:errorcluster, "RobotDriveDevRef"=w109:T16)  [unwired: 6 out]
              n79 = call <vilib>:"WPI_RobotDriveDelayAndUpdateSafety.vi"("error in (no error)"=w108, "Delay (s)"=1.0, "RobotDriveDevRef"=w109) -> ()  [unwired: 7 in, 2 out]
            }
            frame True {
              w146 = 0.0 ("X axis value")
              # "search for hook turns  to find the hook"
              # "Should be 40 in\nsetting 0 for testing"
              n80 = call "Reset Gyro.vi"() -> ("error out"=w153:errorcluster)  [unwired: 11 in]
              n81 = call "Encoder Reset.vi"("error in (no error)"=w153) -> ("error out"=w155:errorcluster)  [unwired: 10 in]
              n82 = call <vilib>:"WPI_RobotDriveRefNum Registry Get.vi"("error in (no error)"=w155, "refnum name"="Left and Right Motors") -> ("error out"=w152:errorcluster, "RobotDriveDevRef"=w154:T16)  [unwired: 8 out]
              n83 = call "drive forward.vi"("error in (no error)"=w152, "forward"=TRUE, "desired distance"=95.0, "RobotDriveDevRef in"=w154) -> ("error out"=w144:errorcluster, "RobotDriveDevRef out"=w145:T16)  [unwired: 6 in]
              n84 = call-poly <vilib>:"WPI_RobotDriveArcadeDrive.vi"("error in (no error)"=w144, "Y axis value"=w146, "X axis value"=w146, "RobotDriveDevRef"=w145) -> ("error out"=w148:errorcluster, "RobotDriveDevRef"=w149:T16)  [unwired: 6 out]
              n85 = call <vilib>:"WPI_RobotDriveDelayAndUpdateSafety.vi"("error in (no error)"=w148, "Delay (s)"=1.0, "RobotDriveDevRef"=w149) -> ("error out"=w142:errorcluster, "RobotDriveDevRef 2"=w143:T16)  [unwired: 7 in]
              n86 = call "turning with gyro left.vi"("desired angle"=45.0, "error in (no error)"=w142, "RobotDriveDevRef"=w143) -> ("error out"=w139:errorcluster, "RobotDriveDevRef 2"=w140:T16)  [unwired: 7 in]
              n87 = call "Auto3.vi"("RobotDriveDevRef"=w140, "error in (no error)"=w139) -> ()  [unwired: 6 in, 8 out]
            }
          }
        }
        frame "1", Default {
          n88 = call-poly <vilib>:"NT Read Value.vi"("Default Value"=FALSE, "Name"="partial auto") -> ("Boolean"=w157:bool)  [unwired: 8 in, 1 out]
          n89 = case shown="False" w157 {
            frame False {
              w163 = 0.0 ("X axis value")
              w174 = 0.0 ("X axis value")
              w181 = 0.0 ("X axis value")
              # "search for hook turns  to find the hook"
              # "Should be 40 in\nsetting 0 for testing"
              n90 = call "Reset Gyro.vi"() -> ("error out"=w188:errorcluster)  [unwired: 11 in]
              n91 = call "Encoder Reset.vi"("error in (no error)"=w188) -> ("error out"=w190:errorcluster)  [unwired: 10 in]
              n92 = call <vilib>:"WPI_RobotDriveRefNum Registry Get.vi"("error in (no error)"=w190, "refnum name"="Left and Right Motors") -> ("error out"=w187:errorcluster, "RobotDriveDevRef"=w189:T16)  [unwired: 8 out]
              n93 = call "drive forward.vi"("error in (no error)"=w187, "forward"=TRUE, "desired distance"=95.0, "RobotDriveDevRef in"=w189) -> ("error out"=w179:errorcluster, "RobotDriveDevRef out"=w180:T16)  [unwired: 6 in]
              n94 = call-poly <vilib>:"WPI_RobotDriveArcadeDrive.vi"("error in (no error)"=w179, "Y axis value"=w181, "X axis value"=w181, "RobotDriveDevRef"=w180) -> ("error out"=w183:errorcluster, "RobotDriveDevRef"=w184:T16)  [unwired: 6 out]
              n95 = call <vilib>:"WPI_RobotDriveDelayAndUpdateSafety.vi"("error in (no error)"=w183, "Delay (s)"=1.0, "RobotDriveDevRef"=w184) -> ("error out"=w177:errorcluster, "RobotDriveDevRef 2"=w178:T16)  [unwired: 7 in]
              n96 = call "turning with gyro.vi"("desired angle"=45.0, "error in (no error)"=w177, "RobotDriveDevRef"=w178) -> ("error out"=w171:errorcluster, "RobotDriveDevRef 2"=w175:T16)  [unwired: 7 in]
              n97 = call-poly <vilib>:"WPI_RobotDriveArcadeDrive.vi"("error in (no error)"=w171, "Y axis value"=w174, "X axis value"=w174, "RobotDriveDevRef"=w175) -> ("error out"=w172:errorcluster, "RobotDriveDevRef"=w173:T16)  [unwired: 6 out]
              n98 = call <vilib>:"WPI_RobotDriveDelayAndUpdateSafety.vi"("error in (no error)"=w172, "Delay (s)"=1.0, "RobotDriveDevRef"=w173) -> ("error out"=w169:errorcluster, "RobotDriveDevRef 2"=w168:T16)  [unwired: 7 in]
              n99 = call "drive forward.vi"("error in (no error)"=w169, "forward"=TRUE, "desired distance"=25.0, "RobotDriveDevRef in"=w168) -> ("error out"=w164:errorcluster, "RobotDriveDevRef out"=w165:T16)  [unwired: 6 in]
              n100 = call-poly <vilib>:"WPI_RobotDriveArcadeDrive.vi"("error in (no error)"=w164, "Y axis value"=w163, "X axis value"=w163, "RobotDriveDevRef"=w165) -> ("error out"=w161:errorcluster, "RobotDriveDevRef"=w162:T16)  [unwired: 6 out]
              n101 = call <vilib>:"WPI_RobotDriveDelayAndUpdateSafety.vi"("error in (no error)"=w161, "Delay (s)"=1.0, "RobotDriveDevRef"=w162) -> ()  [unwired: 7 in, 2 out]
            }
            frame True {
              w199 = 0.0 ("X axis value")
              # "search for hook turns  to find the hook"
              # "Should be 40 in\nsetting 0 for testing"
              n102 = call "Reset Gyro.vi"() -> ("error out"=w206:errorcluster)  [unwired: 11 in]
              n103 = call "Encoder Reset.vi"("error in (no error)"=w206) -> ("error out"=w208:errorcluster)  [unwired: 10 in]
              n104 = call <vilib>:"WPI_RobotDriveRefNum Registry Get.vi"("error in (no error)"=w208, "refnum name"="Left and Right Motors") -> ("error out"=w205:errorcluster, "RobotDriveDevRef"=w207:T16)  [unwired: 8 out]
              n105 = call "drive forward.vi"("error in (no error)"=w205, "forward"=TRUE, "desired distance"=95.0, "RobotDriveDevRef in"=w207) -> ("error out"=w197:errorcluster, "RobotDriveDevRef out"=w198:T16)  [unwired: 6 in]
              n106 = call-poly <vilib>:"WPI_RobotDriveArcadeDrive.vi"("error in (no error)"=w197, "Y axis value"=w199, "X axis value"=w199, "RobotDriveDevRef"=w198) -> ("error out"=w201:errorcluster, "RobotDriveDevRef"=w202:T16)  [unwired: 6 out]
              n107 = call <vilib>:"WPI_RobotDriveDelayAndUpdateSafety.vi"("error in (no error)"=w201, "Delay (s)"=1.0, "RobotDriveDevRef"=w202) -> ("error out"=w195:errorcluster, "RobotDriveDevRef 2"=w196:T16)  [unwired: 7 in]
              n108 = call "turning with gyro.vi"("desired angle"=45.0, "error in (no error)"=w195, "RobotDriveDevRef"=w196) -> ("error out"=w192:errorcluster, "RobotDriveDevRef 2"=w193:T16)  [unwired: 7 in]
              n109 = call "Auto3.vi"("RobotDriveDevRef"=w193, "error in (no error)"=w192) -> ()  [unwired: 6 in, 8 out]
            }
          }
        }
      }
    }
  }
  n110 = disable-structure shown="Disabled" {
    frame Disabled {
      n111 = case shown="True" {
        selector: _ -> [_ _]
        frame False {
        }
        frame True {
          w258 = 0.0 ("X axis value")
          w269 = 0.0 ("X axis value")
          w276 = 0.0 ("X axis value")
          # "search for hook turns  to find the hook"
          # "Should be 40 in\nsetting 0 for testing"
          n112 = call "Reset Gyro.vi"() -> ("error out"=w283:errorcluster)  [unwired: 11 in]
          n113 = call "Encoder Reset.vi"("error in (no error)"=w283) -> ("error out"=w285:errorcluster)  [unwired: 10 in]
          n114 = call <vilib>:"WPI_RobotDriveRefNum Registry Get.vi"("error in (no error)"=w285, "refnum name"="Left and Right Motors") -> ("error out"=w282:errorcluster, "RobotDriveDevRef"=w284:T16)  [unwired: 8 out]
          n115 = call "drive forward.vi"("error in (no error)"=w282, "forward"=TRUE, "desired distance"=95.0, "RobotDriveDevRef in"=w284) -> ("error out"=w274:errorcluster, "RobotDriveDevRef out"=w275:T16)  [unwired: 6 in]
          n116 = call-poly <vilib>:"WPI_RobotDriveArcadeDrive.vi"("error in (no error)"=w274, "Y axis value"=w276, "X axis value"=w276, "RobotDriveDevRef"=w275) -> ("error out"=w278:errorcluster, "RobotDriveDevRef"=w279:T16)  [unwired: 6 out]
          n117 = call <vilib>:"WPI_RobotDriveDelayAndUpdateSafety.vi"("error in (no error)"=w278, "Delay (s)"=1.0, "RobotDriveDevRef"=w279) -> ("error out"=w272:errorcluster, "RobotDriveDevRef 2"=w273:T16)  [unwired: 7 in]
          n118 = call "turning with gyro.vi"("desired angle"=45.0, "error in (no error)"=w272, "RobotDriveDevRef"=w273) -> ("error out"=w266:errorcluster, "RobotDriveDevRef 2"=w270:T16)  [unwired: 7 in]
          n119 = call-poly <vilib>:"WPI_RobotDriveArcadeDrive.vi"("error in (no error)"=w266, "Y axis value"=w269, "X axis value"=w269, "RobotDriveDevRef"=w270) -> ("error out"=w267:errorcluster, "RobotDriveDevRef"=w268:T16)  [unwired: 6 out]
          n120 = call <vilib>:"WPI_RobotDriveDelayAndUpdateSafety.vi"("error in (no error)"=w267, "Delay (s)"=1.0, "RobotDriveDevRef"=w268) -> ("error out"=w264:errorcluster, "RobotDriveDevRef 2"=w263:T16)  [unwired: 7 in]
          n121 = call "drive forward.vi"("error in (no error)"=w264, "forward"=TRUE, "desired distance"=25.0, "RobotDriveDevRef in"=w263) -> ("error out"=w259:errorcluster, "RobotDriveDevRef out"=w260:T16)  [unwired: 6 in]
          n122 = call-poly <vilib>:"WPI_RobotDriveArcadeDrive.vi"("error in (no error)"=w259, "Y axis value"=w258, "X axis value"=w258, "RobotDriveDevRef"=w260) -> ("error out"=w256:errorcluster, "RobotDriveDevRef"=w257:T16)  [unwired: 6 out]
          n123 = call <vilib>:"WPI_RobotDriveDelayAndUpdateSafety.vi"("error in (no error)"=w256, "Delay (s)"=1.0, "RobotDriveDevRef"=w257) -> ()  [unwired: 7 in, 2 out]
        }
      }
      n124 = case shown="True" {
        selector: _ -> [_ _]
        frame False {
        }
        frame True {
          w244 = 0.0 ("X axis value")
          # "Should be 40 in\nsetting 0 for testing"
          n125 = call "Reset Gyro.vi"() -> ("error out"=w251:errorcluster)  [unwired: 11 in]
          n126 = call "Encoder Reset.vi"("error in (no error)"=w251) -> ("error out"=w253:errorcluster)  [unwired: 10 in]
          n127 = call <vilib>:"WPI_RobotDriveRefNum Registry Get.vi"("error in (no error)"=w253, "refnum name"="Left and Right Motors") -> ("error out"=w250:errorcluster, "RobotDriveDevRef"=w252:T16)  [unwired: 8 out]
          n128 = call "drive forward.vi"("error in (no error)"=w250, "forward"=TRUE, "desired distance"=60.0, "RobotDriveDevRef in"=w252) -> ("error out"=w242:errorcluster, "RobotDriveDevRef out"=w243:T16)  [unwired: 6 in]
          n129 = call-poly <vilib>:"WPI_RobotDriveArcadeDrive.vi"("error in (no error)"=w242, "Y axis value"=w244, "X axis value"=w244, "RobotDriveDevRef"=w243) -> ("error out"=w246:errorcluster, "RobotDriveDevRef"=w247:T16)  [unwired: 6 out]
          n130 = call <vilib>:"WPI_RobotDriveDelayAndUpdateSafety.vi"("error in (no error)"=w246, "Delay (s)"=1.0, "RobotDriveDevRef"=w247) -> ()  [unwired: 7 in, 2 out]
        }
      }
      n131 = case shown="True" {
        selector: _ -> [_ _]
        frame False {
        }
        frame True {
          w213 = 0.0 ("X axis value")
          w224 = 0.0 ("X axis value")
          w231 = 0.0 ("X axis value")
          # "search for hook turns  to find the hook"
          # "Should be 40 in\nsetting 0 for testing"
          n132 = call "Reset Gyro.vi"() -> ("error out"=w238:errorcluster)  [unwired: 11 in]
          n133 = call "Encoder Reset.vi"("error in (no error)"=w238) -> ("error out"=w240:errorcluster)  [unwired: 10 in]
          n134 = call <vilib>:"WPI_RobotDriveRefNum Registry Get.vi"("error in (no error)"=w240, "refnum name"="Left and Right Motors") -> ("error out"=w237:errorcluster, "RobotDriveDevRef"=w239:T16)  [unwired: 8 out]
          n135 = call "drive forward.vi"("error in (no error)"=w237, "forward"=TRUE, "desired distance"=95.0, "RobotDriveDevRef in"=w239) -> ("error out"=w229:errorcluster, "RobotDriveDevRef out"=w230:T16)  [unwired: 6 in]
          n136 = call-poly <vilib>:"WPI_RobotDriveArcadeDrive.vi"("error in (no error)"=w229, "Y axis value"=w231, "X axis value"=w231, "RobotDriveDevRef"=w230) -> ("error out"=w233:errorcluster, "RobotDriveDevRef"=w234:T16)  [unwired: 6 out]
          n137 = call <vilib>:"WPI_RobotDriveDelayAndUpdateSafety.vi"("error in (no error)"=w233, "Delay (s)"=1.0, "RobotDriveDevRef"=w234) -> ("error out"=w227:errorcluster, "RobotDriveDevRef 2"=w228:T16)  [unwired: 7 in]
          n138 = call "turning with gyro left.vi"("desired angle"=45.0, "error in (no error)"=w227, "RobotDriveDevRef"=w228) -> ("error out"=w221:errorcluster, "RobotDriveDevRef 2"=w225:T16)  [unwired: 7 in]
          n139 = call-poly <vilib>:"WPI_RobotDriveArcadeDrive.vi"("error in (no error)"=w221, "Y axis value"=w224, "X axis value"=w224, "RobotDriveDevRef"=w225) -> ("error out"=w222:errorcluster, "RobotDriveDevRef"=w223:T16)  [unwired: 6 out]
          n140 = call <vilib>:"WPI_RobotDriveDelayAndUpdateSafety.vi"("error in (no error)"=w222, "Delay (s)"=1.0, "RobotDriveDevRef"=w223) -> ("error out"=w219:errorcluster, "RobotDriveDevRef 2"=w218:T16)  [unwired: 7 in]
          n141 = call "drive forward.vi"("error in (no error)"=w219, "forward"=TRUE, "desired distance"=25.0, "RobotDriveDevRef in"=w218) -> ("error out"=w214:errorcluster, "RobotDriveDevRef out"=w215:T16)  [unwired: 6 in]
          n142 = call-poly <vilib>:"WPI_RobotDriveArcadeDrive.vi"("error in (no error)"=w214, "Y axis value"=w213, "X axis value"=w213, "RobotDriveDevRef"=w215) -> ("error out"=w211:errorcluster, "RobotDriveDevRef"=w212:T16)  [unwired: 6 out]
          n143 = call <vilib>:"WPI_RobotDriveDelayAndUpdateSafety.vi"("error in (no error)"=w211, "Delay (s)"=1.0, "RobotDriveDevRef"=w212) -> ()  [unwired: 7 in, 2 out]
        }
      }
    }
    frame Enabled {
    }
  }
  n144 = disable-structure shown="Enabled" {
    frame Disabled {
      # "This tells you the autonomous selected\nfrom the dashboard"
      # "Every 20ms, report that we are running autonomous\ncode. Loop will abort the same time as the VI."
      # "Use time and/or sensors to control how the robot drives."
      # "This tells you the driver position\nand alliance color"
      n145 = while {
        stop <- FALSE stop-if-true
        n146 = Wait (ms)(milliseconds to wait=u32 20) -> ()  [unwired: 1 out]
        n147 = call <vilib>:"WPI_DriverStationReport Robot Code State.vi"("Autonomous"=TRUE) -> ()  [unwired: 10 in, 1 out]
      }
      n148 = call-poly <vilib>:"NT Read Value.vi"("Name"="Auto Selector") -> ("String"=w289:string)  [unwired: 9 in, 1 out]
      n149 = call <vilib>:"WPI_DriverStationGet Alliance Info.vi"() -> ("Position"=w288:T15)  [unwired: 11 out]
      n150 = case shown="Default" w289 {
        selector: w289 -> [_ _ w320]
        tunnel: w288 -> [_ _ _]
        frame "Alternative 1" {
          # "This sample code describes robot movements in an array. You can extend it to control other motors\non your robot. You can also use file I/O to move the data to a text file."
          n151 = call <vilib>:"WPI_RobotDriveRefNum Registry Get.vi"("refnum name"="Left and Right Motors") -> ("RobotDriveDevRef"=w291:T16)  [unwired: 1 in, 9 out]
          n152 = for {
            shift-right: [w299] -> _
            shift-left: w291 -> [w300]
            tunnel: "Array of robot movements 2" -> [w295] mode=indexing
            n153 = Unbundle By Name(w295) -> ("X Joystick Value"=w298:dbl, "Y Joystick Value"=w297:dbl, "Delay (sec)"=w296:dbl)  [unwired: 1 out]
            n154 = call-poly <vilib>:"WPI_RobotDriveArcadeDrive.vi"("Y axis value"=w297, "X axis value"=w298, "RobotDriveDevRef"=w300) -> ("Motor Values"=w293:dbl[], "RobotDriveDevRef"=w301:T16)  [unwired: 1 in, 6 out]
            n155 = call <vilib>:"WPI_RobotDriveDelayAndUpdateSafety.vi"("Delay (s)"=w296, "RobotDriveDevRef"=w301) -> ("RobotDriveDevRef 2"=w299:T16)  [unwired: 8 in, 1 out]
            n156 = call-poly <vilib>:"NT Write Value.vi"("Numeric Array"=w293, "Name"="RobotDrive Motors") -> ()  [unwired: 9 in, 1 out]
            "Current Movement, for debugging 2" <- w295
          }
        }
        frame "Alternative 2" {
          w303 = "RobotDrive Motors" ("Name")
          # "This is some simple sample code to drive your robot curving one direction and then the other."
          # "stand still"
          # "other way for 0.5 second"
          # "turn for 1 second"
          n157 = call <vilib>:"WPI_RobotDriveRefNum Registry Get.vi"("refnum name"="Left and Right Motors") -> ("RobotDriveDevRef"=w319:T16)  [unwired: 1 in, 9 out]
          n158 = call-poly <vilib>:"WPI_RobotDriveArcadeDrive.vi"("Y axis value"=0.5 ("X axis value"), "X axis value"=-0.25, "RobotDriveDevRef"=w319) -> ("Motor Values"=w302:dbl[], "RobotDriveDevRef"=w312:T16)  [unwired: 1 in, 6 out]
          n159 = call <vilib>:"WPI_RobotDriveDelayAndUpdateSafety.vi"("Delay (s)"=1.0, "RobotDriveDevRef"=w312) -> ("RobotDriveDevRef 2"=w313:T16)  [unwired: 8 in, 1 out]
          n160 = call-poly <vilib>:"WPI_RobotDriveArcadeDrive.vi"("Y axis value"=-0.25 ("X axis value"), "X axis value"=0.5, "RobotDriveDevRef"=w313) -> ("Motor Values"=w304:dbl[], "RobotDriveDevRef"=w314:T16)  [unwired: 1 in, 6 out]
          n161 = call <vilib>:"WPI_RobotDriveDelayAndUpdateSafety.vi"("Delay (s)"=0.5, "RobotDriveDevRef"=w314) -> ("RobotDriveDevRef 2"=w315:T16)  [unwired: 8 in, 1 out]
          n162 = call-poly <vilib>:"NT Write Value.vi"("Numeric Array"=w302, "Name"=w303) -> ()  [unwired: 9 in, 1 out]
          n163 = call-poly <vilib>:"NT Write Value.vi"("Numeric Array"=w304, "Name"=w303) -> ()  [unwired: 9 in, 1 out]
          n164 = call-poly <vilib>:"WPI_RobotDriveArcadeDrive.vi"("Y axis value"=0.0 ("X axis value"), "X axis value"=0.0, "RobotDriveDevRef"=w315) -> ("Motor Values"=w305:dbl[])  [unwired: 1 in, 7 out]
          n165 = call-poly <vilib>:"NT Write Value.vi"("Numeric Array"=w305, "Name"=w303) -> ()  [unwired: 9 in, 1 out]
        }
        frame Default {
          n166 = case shown="\"True\"" w320 {
            frame "False", Default {
            }
            frame "True" {
              w333 = FPGA_DIOChannel."DIO 1"  # B Channel
              w332 = FPGA_DIOChannel."DIO 0"  # A Channel
              w346 = FPGA_DIOChannel."DIO 1"  # B Channel
              w345 = FPGA_DIOChannel."DIO 0"  # A Channel
              w357 = FPGA_DIOChannel."DIO 1"  # B Channel
              w356 = FPGA_DIOChannel."DIO 0"  # A Channel
              w369 = FPGA_DIOChannel."DIO 1"  # B Channel
              w368 = FPGA_DIOChannel."DIO 0"  # A Channel
              w381 = FPGA_DIOChannel."DIO 1"  # B Channel
              w380 = FPGA_DIOChannel."DIO 0"  # A Channel
              w393 = FPGA_DIOChannel."DIO 1"  # B Channel
              w392 = FPGA_DIOChannel."DIO 0"  # A Channel
              w404 = FPGA_DIOChannel."DIO 1"  # B Channel
              w403 = FPGA_DIOChannel."DIO 0"  # A Channel
              (unwired) 0.0 ("Distance")
              # "in inches"
              # "in inches"
              # "in inches"
              # "in inches"
              # "in inches"
              # "in inches"
              # "in inches"
              n167 = call <vilib>:"WPI_DigitalInputOpen.vi"("DIO Channel"=w403) -> ("DigitalInputDevRef"=w400:T4)  [unwired: 1 in, 9 out]
              n168 = call <vilib>:"WPI_DigitalInputOpen.vi"("DIO Channel"=w404) -> ("DigitalInputDevRef"=w401:T4)  [unwired: 1 in, 9 out]
              n169 = call-poly <vilib>:"WPI_CounterToDigitalSource.vi"("DigitalInputDevRef"=w400) -> ("Digital Source"=w321:T5)  [unwired: 6 out]
              n170 = call-poly <vilib>:"WPI_CounterToDigitalSource.vi"("DigitalInputDevRef"=w401) -> ("Digital Source"=w402:T5)  [unwired: 6 out]
              n171 = call <vilib>:"WPI_EncoderOpen.vi"("DistancePerCount"=18.84955592153876, "BSource"=w402, "ASource"=w321) -> ("error out"=w397:errorcluster, "EncoderDevRef"=w398:T9)  [unwired: 5 in, 2 out]
              n172 = call <vilib>:"WPI_EncoderGet.vi"("error in (no error)"=w397, "EncoderDevRef"=w398) -> ("Distance"=w396:dbl)  [unwired: 4 in, 5 out]
              n173 = call <vilib>:"WPI_RobotDriveRefNum Registry Get.vi"("refnum name"="Left Right Motors") -> ("RobotDriveDevRef"=w423:T16)  [unwired: 9 in, 1 out]
              n174 = Equal?(x=w396, y=100.0) -> (x = y?=w394:bool)
              n175 = case shown="True" w394 {
                tunnel: w423 -> [w453 w457]
                tunnel: [w453 w454] -> w422
                frame False {
                }
                frame True {
                  n176 = call-poly <vilib>:"WPI_RobotDriveArcadeDrive.vi"("Y axis value"=0.05, "X axis value"=0.0, "RobotDriveDevRef"=w457) -> ("RobotDriveDevRef"=w454:T16)  [unwired: 6 in, 2 out]
                }
              }
              n177 = call <vilib>:"WPI_DigitalInputOpen.vi"("DIO Channel"=w392) -> ("DigitalInputDevRef"=w389:T4)  [unwired: 1 in, 9 out]
              n178 = call <vilib>:"WPI_DigitalInputOpen.vi"("DIO Channel"=w393) -> ("DigitalInputDevRef"=w390:T4)  [unwired: 1 in, 9 out]
              n179 = call-poly <vilib>:"WPI_CounterToDigitalSource.vi"("DigitalInputDevRef"=w389) -> ("Digital Source"=w388:T5)  [unwired: 6 out]
              n180 = call-poly <vilib>:"WPI_CounterToDigitalSource.vi"("DigitalInputDevRef"=w390) -> ("Digital Source"=w391:T5)  [unwired: 6 out]
              n181 = call <vilib>:"WPI_EncoderOpen.vi"("DistancePerCount"=18.84955592153876, "BSource"=w391, "ASource"=w388) -> ("error out"=w385:errorcluster, "EncoderDevRef"=w386:T9)  [unwired: 5 in, 2 out]
              n182 = call <vilib>:"WPI_EncoderGet.vi"("error in (no error)"=w385, "EncoderDevRef"=w386) -> ("Distance"=w384:dbl)  [unwired: 4 in, 5 out]
              n183 = call <vilib>:"WPI_RobotDriveDelayAndUpdateSafety.vi"("Delay (s)"=0.07, "RobotDriveDevRef"=w422) -> ("RobotDriveDevRef 2"=w418:T16)  [unwired: 8 in, 1 out]
              n184 = Equal?(x=w384, y=100.0) -> (x = y?=w382:bool)
              n185 = case shown="True" w382 {
                tunnel: w418 -> [w448 w452]
                tunnel: [w448 w449] -> w420
                frame False {
                }
                frame True {
                  n186 = call-poly <vilib>:"WPI_RobotDriveArcadeDrive.vi"("Y axis value"=0.15, "X axis value"=0.0, "RobotDriveDevRef"=w452) -> ("RobotDriveDevRef"=w449:T16)  [unwired: 6 in, 2 out]
                }
              }
              n187 = call <vilib>:"WPI_DigitalInputOpen.vi"("DIO Channel"=w380) -> ("DigitalInputDevRef"=w377:T4)  [unwired: 1 in, 9 out]
              n188 = call <vilib>:"WPI_DigitalInputOpen.vi"("DIO Channel"=w381) -> ("DigitalInputDevRef"=w378:T4)  [unwired: 1 in, 9 out]
              n189 = call-poly <vilib>:"WPI_CounterToDigitalSource.vi"("DigitalInputDevRef"=w377) -> ("Digital Source"=w376:T5)  [unwired: 6 out]
              n190 = call-poly <vilib>:"WPI_CounterToDigitalSource.vi"("DigitalInputDevRef"=w378) -> ("Digital Source"=w379:T5)  [unwired: 6 out]
              n191 = call <vilib>:"WPI_EncoderOpen.vi"("DistancePerCount"=18.84955592153876, "BSource"=w379, "ASource"=w376) -> ("error out"=w373:errorcluster, "EncoderDevRef"=w374:T9)  [unwired: 5 in, 2 out]
              n192 = call <vilib>:"WPI_EncoderGet.vi"("error in (no error)"=w373, "EncoderDevRef"=w374) -> ("Distance"=w372:dbl)  [unwired: 4 in, 5 out]
              n193 = call <vilib>:"WPI_RobotDriveDelayAndUpdateSafety.vi"("Delay (s)"=0.1, "RobotDriveDevRef"=w420) -> ("RobotDriveDevRef 2"=w415:T16)  [unwired: 8 in, 1 out]
              n194 = Equal?(x=w372, y=100.0) -> (x = y?=w370:bool)
              n195 = case shown="True" w370 {
                tunnel: w415 -> [w443 w447]
                tunnel: [w443 w444] -> w417
                frame False {
                }
                frame True {
                  n196 = call-poly <vilib>:"WPI_RobotDriveArcadeDrive.vi"("Y axis value"=0.3, "X axis value"=0.0, "RobotDriveDevRef"=w447) -> ("RobotDriveDevRef"=w444:T16)  [unwired: 6 in, 2 out]
                }
              }
              n197 = call <vilib>:"WPI_DigitalInputOpen.vi"("DIO Channel"=w368) -> ("DigitalInputDevRef"=w365:T4)  [unwired: 1 in, 9 out]
              n198 = call <vilib>:"WPI_DigitalInputOpen.vi"("DIO Channel"=w369) -> ("DigitalInputDevRef"=w366:T4)  [unwired: 1 in, 9 out]
              n199 = call-poly <vilib>:"WPI_CounterToDigitalSource.vi"("DigitalInputDevRef"=w365) -> ("Digital Source"=w364:T5)  [unwired: 6 out]
              n200 = call-poly <vilib>:"WPI_CounterToDigitalSource.vi"("DigitalInputDevRef"=w366) -> ("Digital Source"=w367:T5)  [unwired: 6 out]
              n201 = call <vilib>:"WPI_EncoderOpen.vi"("DistancePerCount"=18.84955592153876, "BSource"=w367, "ASource"=w364) -> ("error out"=w361:errorcluster, "EncoderDevRef"=w362:T9)  [unwired: 5 in, 2 out]
              n202 = call <vilib>:"WPI_EncoderGet.vi"("error in (no error)"=w361, "EncoderDevRef"=w362) -> ("Distance"=w360:dbl)  [unwired: 4 in, 5 out]
              n203 = call <vilib>:"WPI_RobotDriveDelayAndUpdateSafety.vi"("Delay (s)"=0.1, "RobotDriveDevRef"=w417) -> ("RobotDriveDevRef 2"=w413:T16)  [unwired: 8 in, 1 out]
              n204 = Equal?(x=w360, y=100.0) -> (x = y?=w358:bool)
              n205 = case shown="True" w358 {
                tunnel: w413 -> [w438 w442]
                tunnel: [w438 w439] -> w414
                frame False {
                }
                frame True {
                  n206 = call-poly <vilib>:"WPI_RobotDriveArcadeDrive.vi"("Y axis value"=0.5, "X axis value"=0.0, "RobotDriveDevRef"=w442) -> ("RobotDriveDevRef"=w439:T16)  [unwired: 6 in, 2 out]
                }
              }
              n207 = call <vilib>:"WPI_DigitalInputOpen.vi"("DIO Channel"=w356) -> ("DigitalInputDevRef"=w353:T4)  [unwired: 1 in, 9 out]
              n208 = call <vilib>:"WPI_DigitalInputOpen.vi"("DIO Channel"=w357) -> ("DigitalInputDevRef"=w354:T4)  [unwired: 1 in, 9 out]
              n209 = call-poly <vilib>:"WPI_CounterToDigitalSource.vi"("DigitalInputDevRef"=w353) -> ("Digital Source"=w352:T5)  [unwired: 6 out]
              n210 = call-poly <vilib>:"WPI_CounterToDigitalSource.vi"("DigitalInputDevRef"=w354) -> ("Digital Source"=w355:T5)  [unwired: 6 out]
              n211 = call <vilib>:"WPI_EncoderOpen.vi"("DistancePerCount"=18.84955592153876, "BSource"=w355, "ASource"=w352) -> ("error out"=w349:errorcluster, "EncoderDevRef"=w350:T9)  [unwired: 5 in, 2 out]
              n212 = call <vilib>:"WPI_EncoderGet.vi"("error in (no error)"=w349, "EncoderDevRef"=w350) -> ("Distance"=w348:dbl)  [unwired: 4 in, 5 out]
              n213 = call <vilib>:"WPI_RobotDriveDelayAndUpdateSafety.vi"("Delay (s)"=0.1, "RobotDriveDevRef"=w414) -> ("RobotDriveDevRef 2"=w409:T16)  [unwired: 8 in, 1 out]
              n214 = Equal?(x=w348, y=100.0) -> (x = y?=w335:bool)
              n215 = case shown="True" w335 {
                tunnel: w409 -> [w433 w437]
                tunnel: [w433 w434] -> w410
                frame False {
                }
                frame True {
                  n216 = call-poly <vilib>:"WPI_RobotDriveArcadeDrive.vi"("Y axis value"=0.7, "X axis value"=0.0, "RobotDriveDevRef"=w437) -> ("RobotDriveDevRef"=w434:T16)  [unwired: 6 in, 2 out]
                }
              }
              n217 = call <vilib>:"WPI_DigitalInputOpen.vi"("DIO Channel"=w345) -> ("DigitalInputDevRef"=w342:T4)  [unwired: 1 in, 9 out]
              n218 = call <vilib>:"WPI_DigitalInputOpen.vi"("DIO Channel"=w346) -> ("DigitalInputDevRef"=w343:T4)  [unwired: 1 in, 9 out]
              n219 = call-poly <vilib>:"WPI_CounterToDigitalSource.vi"("DigitalInputDevRef"=w342) -> ("Digital Source"=w341:T5)  [unwired: 6 out]
              n220 = call-poly <vilib>:"WPI_CounterToDigitalSource.vi"("DigitalInputDevRef"=w343) -> ("Digital Source"=w344:T5)  [unwired: 6 out]
              n221 = call <vilib>:"WPI_EncoderOpen.vi"("DistancePerCount"=18.84955592153876, "BSource"=w344, "ASource"=w341) -> ("error out"=w338:errorcluster, "EncoderDevRef"=w339:T9)  [unwired: 5 in, 2 out]
              n222 = call <vilib>:"WPI_EncoderGet.vi"("error in (no error)"=w338, "EncoderDevRef"=w339) -> ("Distance"=w337:dbl)  [unwired: 4 in, 5 out]
              n223 = call <vilib>:"WPI_RobotDriveDelayAndUpdateSafety.vi"("Delay (s)"=0.1, "RobotDriveDevRef"=w410) -> ("RobotDriveDevRef 2"=w406:T16)  [unwired: 8 in, 1 out]
              n224 = Equal?(x=w337, y=100.0) -> (x = y?=w334:bool)
              n225 = case shown="True" w334 {
                tunnel: w406 -> [w428 w432]
                tunnel: [w428 w429] -> w407
                frame False {
                }
                frame True {
                  n226 = call-poly <vilib>:"WPI_RobotDriveArcadeDrive.vi"("Y axis value"=0.9, "X axis value"=0.0, "RobotDriveDevRef"=w432) -> ("RobotDriveDevRef"=w429:T16)  [unwired: 6 in, 2 out]
                }
              }
              n227 = call <vilib>:"WPI_DigitalInputOpen.vi"("DIO Channel"=w332) -> ("DigitalInputDevRef"=w329:T4)  [unwired: 1 in, 9 out]
              n228 = call <vilib>:"WPI_DigitalInputOpen.vi"("DIO Channel"=w333) -> ("DigitalInputDevRef"=w330:T4)  [unwired: 1 in, 9 out]
              n229 = call-poly <vilib>:"WPI_CounterToDigitalSource.vi"("DigitalInputDevRef"=w329) -> ("Digital Source"=w328:T5)  [unwired: 6 out]
              n230 = call-poly <vilib>:"WPI_CounterToDigitalSource.vi"("DigitalInputDevRef"=w330) -> ("Digital Source"=w331:T5)  [unwired: 6 out]
              n231 = call <vilib>:"WPI_EncoderOpen.vi"("DistancePerCount"=18.84955592153876, "BSource"=w331, "ASource"=w328) -> ("error out"=w325:errorcluster, "EncoderDevRef"=w326:T9)  [unwired: 5 in, 2 out]
              n232 = call <vilib>:"WPI_EncoderGet.vi"("error in (no error)"=w325, "EncoderDevRef"=w326) -> ("Distance"=w324:dbl)  [unwired: 4 in, 5 out]
              n233 = call <vilib>:"WPI_RobotDriveDelayAndUpdateSafety.vi"("Delay (s)"=0.1, "RobotDriveDevRef"=w407) -> ("RobotDriveDevRef 2"=w405:T16)  [unwired: 8 in, 1 out]
              n234 = Equal?(x=w324, y=100.0) -> (x = y?=w322:bool)
              n235 = case shown="True" w322 {
                tunnel: w405 -> [_ w427]
                frame False {
                }
                frame True {
                  n236 = call-poly <vilib>:"WPI_RobotDriveArcadeDrive.vi"("Y axis value"=0.5, "X axis value"=0.0, "RobotDriveDevRef"=w427) -> ()  [unwired: 6 in, 3 out]
                }
              }
            }
          }
        }
      }
    }
    frame Enabled {
    }
  }
  n237 = Index Array(array=w3, index #1=2 ("index")) -> ()  [unwired: 1 in, 2 out]
  n238 = call-poly <vilib>:"NT Write Value.vi"("Numeric Array"=w3, "Name"="Joystick 0/Axes") -> ()  [unwired: 9 in, 1 out]
